vi "slow_control_2_12.vi"() -> ()   [LabVIEW 2018]
uses:
  4623b864-5764-45c6-9cb2-3e18237880ca.vi
  fa57f61f-0bb9-49ac-92eb-fcb40add4dbb.vi
  499f9cf5-7b15-41ea-951a-8da9be12721d.vi
  <vilib>/DAQmx/read.llb/DAQmx Read (Analog 1D DBL NChan 1Samp).vi
  ffb0d1b3-ef19-4e2e-b36e-7277177ef4b3.vi
  9a1acc8a-69db-4048-9e4c-bb07d66d2422.vi
  <vilib>/DAQmx/create/channels.llb/DAQmx Create Channel (AI-Voltage-Basic).vi
  <vilib>/DAQmx/create/channels.llb/DAQmx Create Channel (AI-Current-Basic).vi
  <vilib>/DAQmx/create/channels.llb/DAQmx Create Channel (AI-Temperature-RTD).vi
  <vilib>/DAQmx/miscellaneous.llb/DAQmx Fill In Error Info.vi
  <vilib>/Utility/file.llb/Read Delimited Spreadsheet (string).vi
  <instrlib>/Lake Shore 335/Lake Shore 335.lvlib
  <instrlib>/CAEN PSM/CAEN PSM.lvlib
  <resource>/objmgr/daqmx.rc
panel:
  out "Heater":dbl
  out "Coldhead":dbl
  out "Cycle number":i32
  out "Alarm state":bool
  out "Timestamp last \nmeasured (UPS)":timestamp
  out "Auto-clear":bool
  in  "Auto-clear data?":bool
  in  "Clear data":bool
  in  "Clear data every N cycles":dbl
  in  "N samples":i32=30
  out "Average Flow (SLPM)":dbl caption="Flow (SLPM)"
  out "CAEN Ch. Names":string[](array[string])
  in  "Cycles to execute":dbl=5.0 format="%#_13g"
  out "Detector Pressure":dbl
  in  "N samples":i32=20
  in  "Allows tabs on \nfront panel":T1(tab)
  in  "Specify up to six temperature sensors inside \nthe detector, separated with a comma.\nNumbers only, single commas!":string="10,11,12,13,14,15"
  out "Valid example:":string="11,12, 13, 15 ,14 "
  in  "Anode ch.":enum16{"1", "2", "3", "4"}(ring)=enum."3"
  in  "CAEN unit selector":enum16{"CAEN 1", "CAEN 2"}(ring)
  in  "Multipliers":dbl[](array[numeric])=[1.0, 1.0, 1.0, 1.0, 1.0, 1.0, 1.0, 1.0]
  in  "Offsets\nsubtracted":dbl[](array[numeric])=[0.0, 0.0, 0.0, 0.0, 0.0, 0.0, 0.0, 0.0]
  in  "Channel Names (9207, ai8:15)":string[](array[string])=["i0", "i1", "i2", "i3", "i4", "i5", "i6", "i7"] caption="\"Other\""
  in  "Flow meter input:":u16(ring)=3 items=["v0", "v1", "v2", "v3", "v4", "v5", "v6", "v7"]
  in  "Detector pressure input:":u16(ring) items=["v0", "v1", "v2", "v3", "v4", "v5", "v6", "v7"]
  in  "Channel Names (9207, ai0:7)":string[](array[string])=["v0", "v1", "v2", "v3", "v4", "v5", "v6", "v7"] caption="\"Other\""
  in  "Multipliers":dbl[](array[numeric])=[1.0, 1.0, 1.0, 1.0, 1.0, 1.0, 1.0, 1.0]
  in  "Offsets\nsubtracted":dbl[](array[numeric])=[0.0, 0.0, 0.0, 0.0, 0.0, 0.0, 0.0, 0.0]
  in  "Voltage channels":tag[](array[tag])=["9207/ai0", "9207/ai1", "9207/ai2", "9207/ai3", "9207/ai4", "9207/ai5", "9207/ai6", "9207/ai7"]
  in  "COM-port CAEN 1":refnum<visa-resource-name>
  in  "COM-port CAEN 2":refnum<visa-resource-name>
  in  "Run lakeshore?":bool
  in  "ID Query":bool
  in  "COM-port LakeShore":refnum<visa-resource-name>
  in  "PID settings":cluster{"P":dbl, "I":dbl, "D":dbl}={"P"=50.0, "I"=20.0, "D"=120.0}
  in  "Setpoint (°C)":dbl=-100.0 format="%.1f"
  in  "Heater range":u16(ring) items=["Off", "Low (On)", "Medium", "High"]
  in  "Current channels":tag[](array[tag])=["9207/ai8", "9207/ai9", "9207/ai10", "9207/ai11", "9207/ai12", "9207/ai13", "9207/ai14", "9207/ai15"]
  in  "Channel Names (CAEN)":string[](array[string])=["PMT 1", "PMT 2", "Anode", "Cathode", "Top gate", "Bottom gate", "Other 1", "Other 2"]
  in  "RTD Type":i32(ring)=10071 items=["Pt3750"=12481, "Pt3851"=10071, "Pt3911"=12482, "Pt3916"=10069, "Pt3920"=10053, "Pt3928"=12483, "Custom"=10137]
  in  "Module 1 channels (slot 1)":tag[](array[tag])=["cDAQ2Mod2/ai0", "cDAQ2Mod2/ai1", "cDAQ2Mod2/ai2", "cDAQ2Mod2/ai3", "cDAQ2Mod2/ai4", "cDAQ2Mod2/ai5", "cDAQ2Mod2/ai6", "cDAQ2Mod2/ai7"]
  in  "Current Excitation Source":i32(ring)=10200 items=["Internal"=10200, "External"=10167, "None"=10230]
  in  "Resistance Configuration":i32(ring)=3 items=["2-Wire"=2, "3-Wire"=3, "4-Wire"=4]
  in  "R (T = 0°C):":dbl=100.0
  in  "B":dbl
  in  "A":dbl
  in  "C":dbl
  in  "Module 2 channels (slot 2)":tag[](array[tag])=["cDAQ2Mod3/ai0", "cDAQ2Mod3/ai1", "cDAQ2Mod3/ai2", "cDAQ2Mod2/ai3", "cDAQ2Mod2/ai4", "cDAQ2Mod3/ai5", "cDAQ2Mod3/ai6", "cDAQ2Mod3/ai7"]
  in  "Shut off heater \nif Alarm is active":bool=TRUE
  in  "Re-save headers":bool
  in  "Resistance Configuration":i32(ring)=2 items=["2-Wire"=2, "3-Wire"=3, "4-Wire"=4]
  in  "Module 3 channels":tag[](array[tag])
  in  "RTD Type":i32(ring)=12481 items=["Pt3750"=12481, "Pt3851"=10071, "Pt3911"=12482, "Pt3916"=10069, "Pt3920"=10053, "Pt3928"=12483, "Custom"=10137]
  in  "R (T = 0°C)":dbl=100.0 format="%0.2f"
  out "PT1000 data":dbl[](array[numeric]) format="%0.2f"
  out "Det. T.":i32[](array[numeric])
  out "9207 (V; A) Converted":dbl[](array[numeric])
  out "9216 #1 (°C)":dbl[](array[numeric])
  out "9216 #2 (°C)":dbl[](array[numeric])
  out "Raw readouts (V, mA)":dbl[](array[numeric]) format="%0.2f"
  out "Det.P input #":i32
  out "Flow input #":i32
  out "PT100 data":dbl[](array[numeric]) format="%0.2f"
  in  "\"Sound\" alarm":bool
  in  "Sound alarm\nFrequency (Hz)":dbl=1680.0
  in  "Send status email now":bool
  out "Email error":i32
  out "source":string
  in  "Number of Bonus lines":i32=1
  out "Names (optional)":string[](array[string])
  in  "Send daily email?":bool=TRUE
  in  "Phone numbers":string[](array[string])
  out "Alarm (or test) message":string
  in  "Alarm\nMaster switch":bool
  in  "Repeat Alarm SMS\nevery N minutes":dbl=15.0
  in  "Test alarm":bool
  out "Warning":bool
  in  "UPS":bool
  in  "UPS Voltage \nLower Threshold":dbl=220.0
  out "String 6":string
  out "String 5":string
  out "String 4":string
  out "String 3":string
  out "String 2":string
  out "String":string
  out "NI mod 2&3 status":bool
  in  "NI mod 2&3":bool
  in  "NI mod 1":bool
  in  "CAEN 2":bool
  in  "CAEN 1":bool
  in  "LakeShore":bool
  out "Det. P. warning":bool
  out "Boolean 6":bool
  out "Boolean 5":bool
  out "Boolean 4":bool
  out "Boolean 3":bool
  out "Boolean 2":bool
  out "Boolean":bool
  in  "T 6":bool
  in  "T 5":bool
  in  "T 4":bool
  in  "T 3":bool
  in  "T 2":bool
  in  "T 1":bool
  in  "Detector Pressure":bool
  in  "Overpressure threshold":dbl
  in  "Underpressure threshold":dbl
  out "Comm. status":bool
  in  "High Temp threshold":dbl format="%#_13g"
  in  "Low Temp threshold":dbl format="%#_13g"
  out "LakeShore status":bool
  out "NI mod1 (P) status":bool
  out "CAEN 1 status":bool
  out "CAEN 2 status":bool
  out "Initialization status":bool
  out "Minimum input voltage measured":dbl
  out "Alarm active 2":bool
  out "SMS error":string
  out "Status email preview":string
  in  "Send status email at time:":string="14:00"
  in  "Email Addresses":string[](array[string])
  in  "return address":string="xamsups@gmail.com"
  in  "Ignore Initialization Errors":bool=TRUE caption="Ignore init. errors?"
  out "NI 9226":errorcluster
  in  "HV Channel status":string="Click the button to request the latest High Voltage channel status."
  out "CAEN 1":T2(array[cluster])
  out "CAEN 2":T2(array[cluster])
  in  "Query HV status":bool
  in  "\"code\"":string
  in  "String 7":string
  out "\"status\"":bool
  in  "\"source\"":string
  out "NI 9216 x2":errorcluster
  out "CAEN 1":errorcluster
  out "CAEN 2":errorcluster
  out "Lakeshore":errorcluster
  out "NI 9207":errorcluster
  out "9207 (ai 8:15, Amperes)":cluster{timestamp[], dbl[]}[](graph)
  in  "Temperature channel selector":u16(ring)=10 items=["10"=10, "11"=11, "12"=12, "13"=13, "14"=14, "15"=15, "Average"=666]
  out "Heater power (%)":cluster{timestamp[], dbl[]}[](graph)
  out "Flow (SLPM)":cluster{timestamp[], dbl[]}[](graph)
  out "9207 (ai 0:7, Volts)":cluster{timestamp[], dbl[]}[](graph)
  out "Phase Diagram":cluster{"X":dbl, "Y":dbl}[](graph)
  out "Temperature (ai 0:15, °C)":cluster{timestamp[], dbl[]}[](graph)
  in  "Pause?":bool
  out "Integrated Flow (SL)":dbl
  in  "Reset?":bool
  out "LakeShore readings":dbl[](array[numeric])
  out "Temp A":dbl
  out "Temp B":dbl
  in  "Temperature Channel Selector":u16(ring) items=["10"=10, "11"=11, "12"=12, "13"=13, "14"=14, "15"=15]
  out "Historical Large Phase Diagram":cluster{dbl[], dbl[]}[](graph)
  out "Large Phase Diagram":cluster{"X":dbl, "Y":dbl}[](graph)
  in  "Temperature Channel Selector":u16(ring)=666 items=["10"=10, "11"=11, "12"=12, "13"=13, "14"=14, "15"=15, "Average"=666]
  in  "Scale.Range:Minimum 8":dbl
  in  "Scale.Range:Maximum 8":dbl=4000.0
  in  "Scale.Range:Minimum 7":dbl
  in  "Scale.Range:Maximum 7":dbl=4000.0
  in  "Scale.Range:Minimum 6":dbl=-3000.0
  in  "Scale.Range:Maximum 6":dbl
  in  "Scale.Range:Minimum 5":dbl
  in  "Scale.Range:Maximum 5":dbl=3000.0
  in  "Scale.Range:Minimum 4":dbl=-5000.0
  in  "Scale.Range:Maximum 4":dbl
  in  "Scale.Range:Maximum 3":dbl=4000.0
  in  "Scale.Range:Minimum 3":dbl
  in  "Scale.Range:Maximum 2":dbl=1000.0
  in  "Scale.Range:Minimum 2":dbl
  out "CAEN 1.1":dbl(knob) scale=0.0..1000.0
  out "CAEN 1.1":string
  in  "Scale.Range:Maximum":dbl=1000.0
  in  "Scale.Range:Minimum":dbl
  out "CAEN 2.3 2":string
  out "CAEN 2.2 2":string
  out "Channel Names":string[](array[string])
  out "CAEN 2.3":dbl(knob) scale=0.0..4000.0
  out "CAEN 2.2":dbl(knob) scale=0.0..4000.0
  out "CAEN 2.1":string
  out "CAEN 2.0":string
  out "CAEN 1.3":string
  out "CAEN 1.2":string
  out "CAEN 1.0":string
  out "Channel Names":string[](array[string])
  in  "Set to zero":bool
  out "CAEN 2.1":dbl(knob)
  out "CAEN 2.0":dbl(knob) scale=0.0..3000.0
  in  "Apply Voltage":bool
  in  "VSet (V)":dbl[](array[numeric])
  in  "IMax (uA)":dbl[](array[numeric])
  in  "VMax (V)":dbl[](array[numeric])
  out "CAEN 1.3":dbl(knob)
  out "CAEN 1.2":dbl(knob) scale=0.0..4000.0
  out "CAEN 1.0":dbl(knob) scale=0.0..1000.0
  out "Vmon (V)":dbl[](array[numeric])
  out "IMon (uA)":dbl[](array[numeric])
  in  "Read CAEN units \nevery N cycles":i16=120
  in  "Reset anode\nperiodically?":bool
  in  "Kill every Y minutes":i32=10
  in  "Keep off for X seconds":i32=10
  out "?":bool
  out "Killed":bool
  out "Restarted":bool
  out "Anode timers":timestamp[](array[timestamp])
  out "Seconds until \nanode autokill":dbl format="%.2g"
  out "Seconds until \nanode reset":dbl format="%.2g"
  in  "Kill voltage":bool
  in  "stop":bool
  out "Voltages":dbl[](array[numeric])
  out "Started up?":bool
  out "TOBA appended":dbl[][](array[numeric])
  in  "Read T every N cycles":i32=2
  out "Time until next cycle":dbl format="%.3g"
  in  "Time per cycle (s)":i32=2 caption="Time Target (s)"
  # "<- Proof of concept for New/Old T + New P"
  # "Moving averages"
  # "NI 9216 Temperature settings"
  # "CAEN settings"
  # "NI 9207 Voltage settings"
  # "If RTD type is custom,\nspecify the Callendar-\nVan Dusen parameters"
  # "Anode connected to:"
  # "Channel:"
  # "NI 9207 Current settings"
  # "Lakeshore settings"
  # "NI 9226 Temperature settings"
  # "Gain (P) (XX.X)"
  # "Reset (I) (XX.X)"
  # "Rate (D) (X.X%)"
  # "Alarm indicators and arms"
  # "Detector Thresholds"
  # "Daily status email"
  # "SMS and sound alarm"
  # "Alarm conditions"
  # "Temperature channels:"
  # "Uninterruptable Power Supply"
  # "Device information"
  # "High Voltage channel status"
  # "How-to"
  # "Data"
  # "Scale:"
  # "to"
  # "to"
  # "Scale:"
  # "Time of last reset"
  # "Time of last reactivation"
  # "to"
  # "Scale:"
  # "to"
  # "Scale:"
  # "Settings"
  # "Scale:"
  # "to"
  # "Scale:"
  # "to"
  # "Scale:"
  # "to"
  # "to"
  # "Scale:"
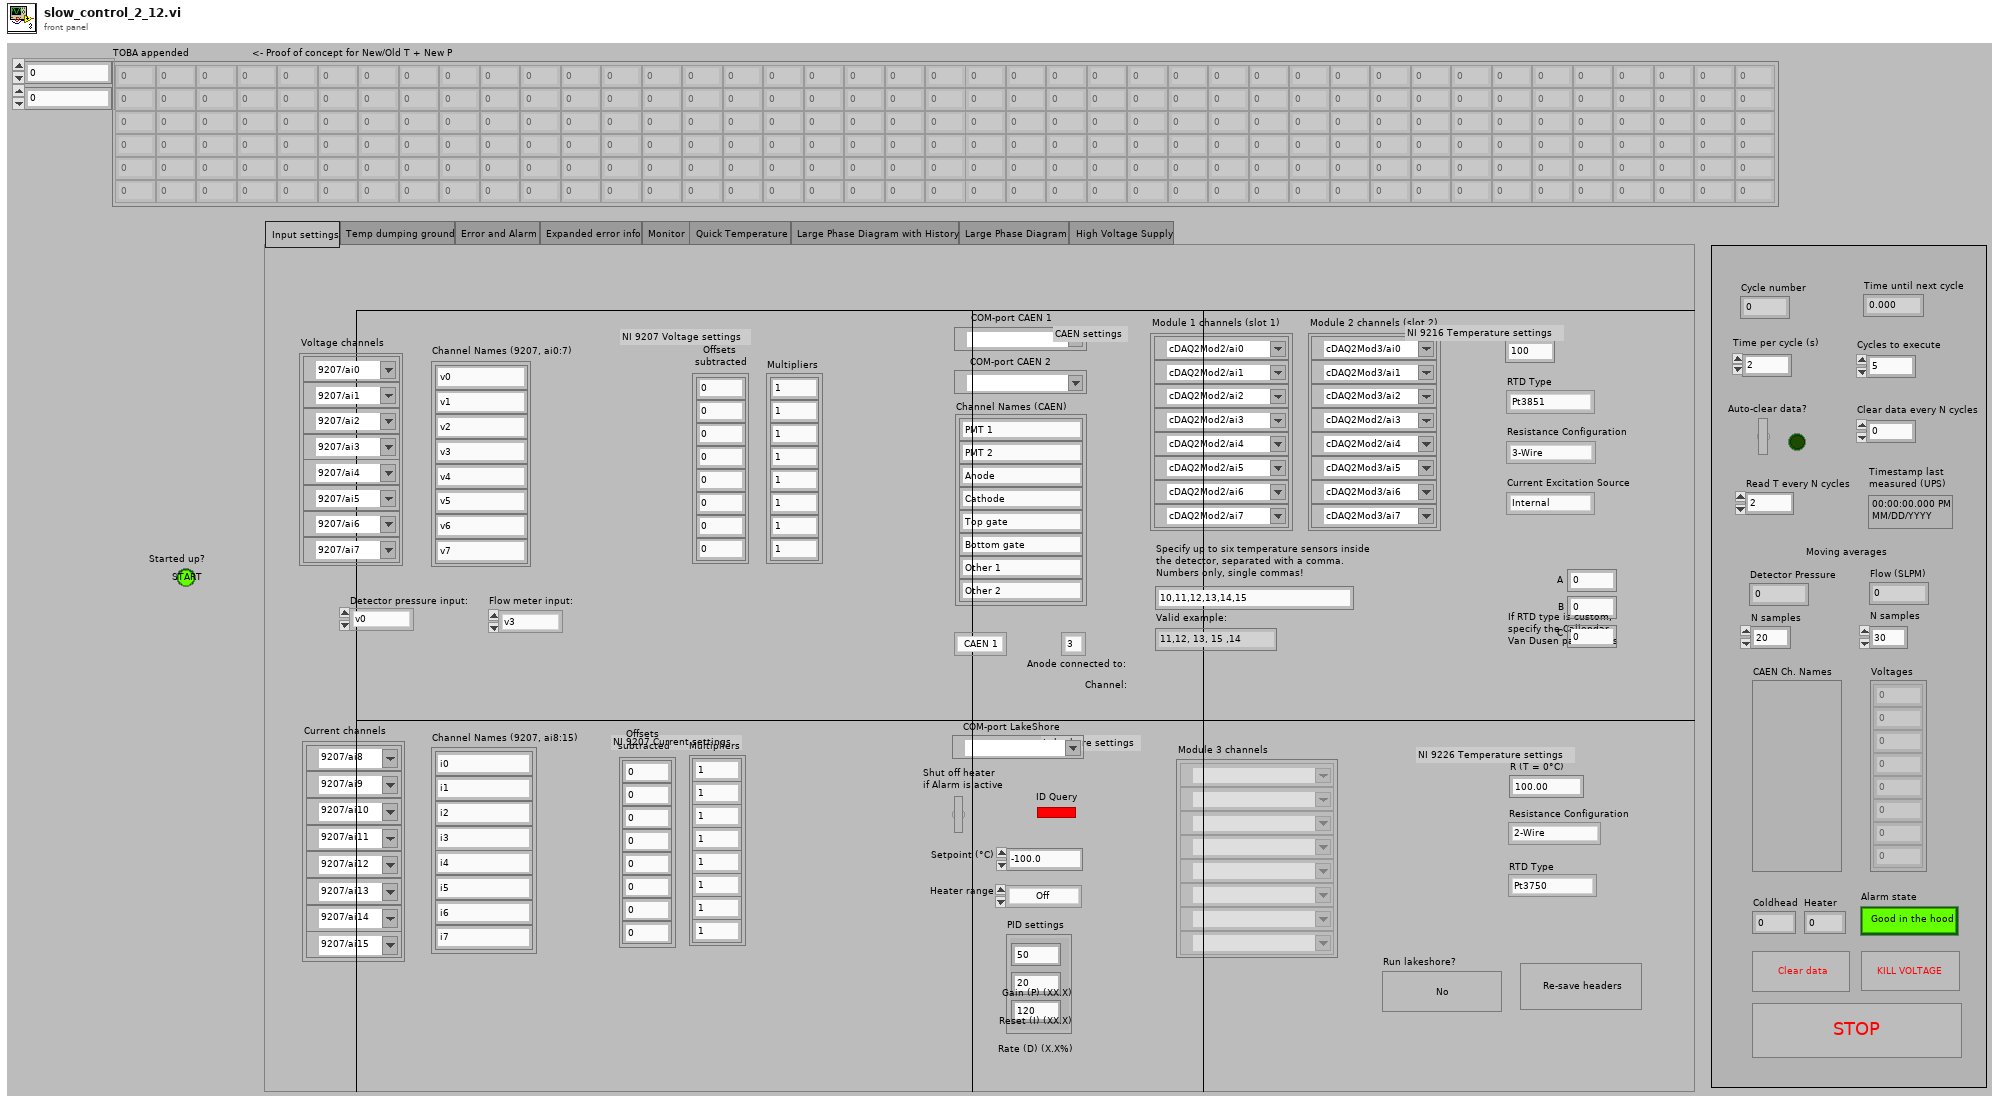
[diagram p1: front panel]
types:
  T1 = enum32{"Input settings", "Temp dumping ground", "Error and Alarm", "Expanded error info", "Monitor", "Quick Temperature", "Large Phase Diagram with History", "Large Phase Diagram", "High Voltage Supply"}
  T2 = cluster{"ON":bool, "RUP":bool, "RDW":bool, "OVC":bool, "OVV":bool, "UNV":bool, "MAXV":bool, "TRIP":bool, "OVP":bool, "OVT":bool, "DIS":bool, "KILL":bool, "ILK":bool, "NOCAL":bool}[]
  T3 = cluster{"Baud Rate":u32, "Parity":u16, "Data Bits":u16, "Stop Bits":u16, "Flow Control":u16}
  T4 = cluster{"task out":refnum<k21>, "error out":errorcluster}
  T5 = cluster{"VISA resource name out":refnum<visa-resource-name>, "error out":errorcluster}
  T6 = cluster{"VISA resource name out":refnum<visa-resource-name>, "Board address":u8, "NChannels":u8}
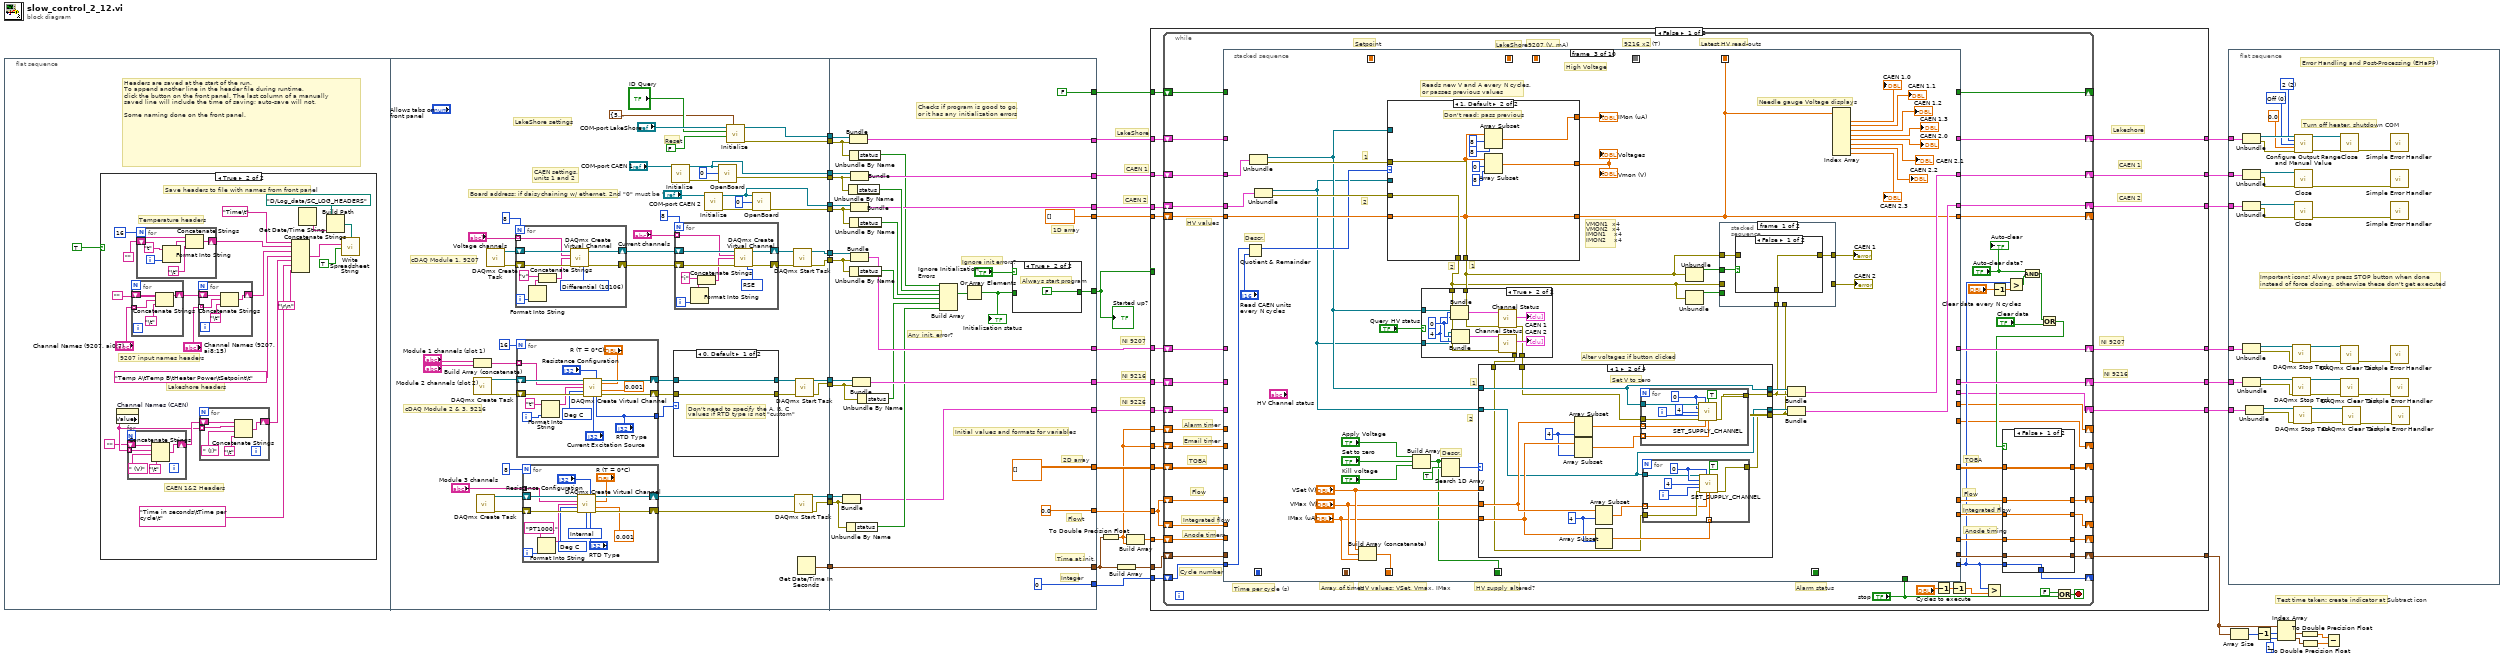
[diagram p0: block diagram]
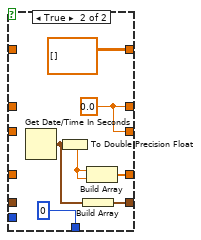
[diagram p2: hidden frame]
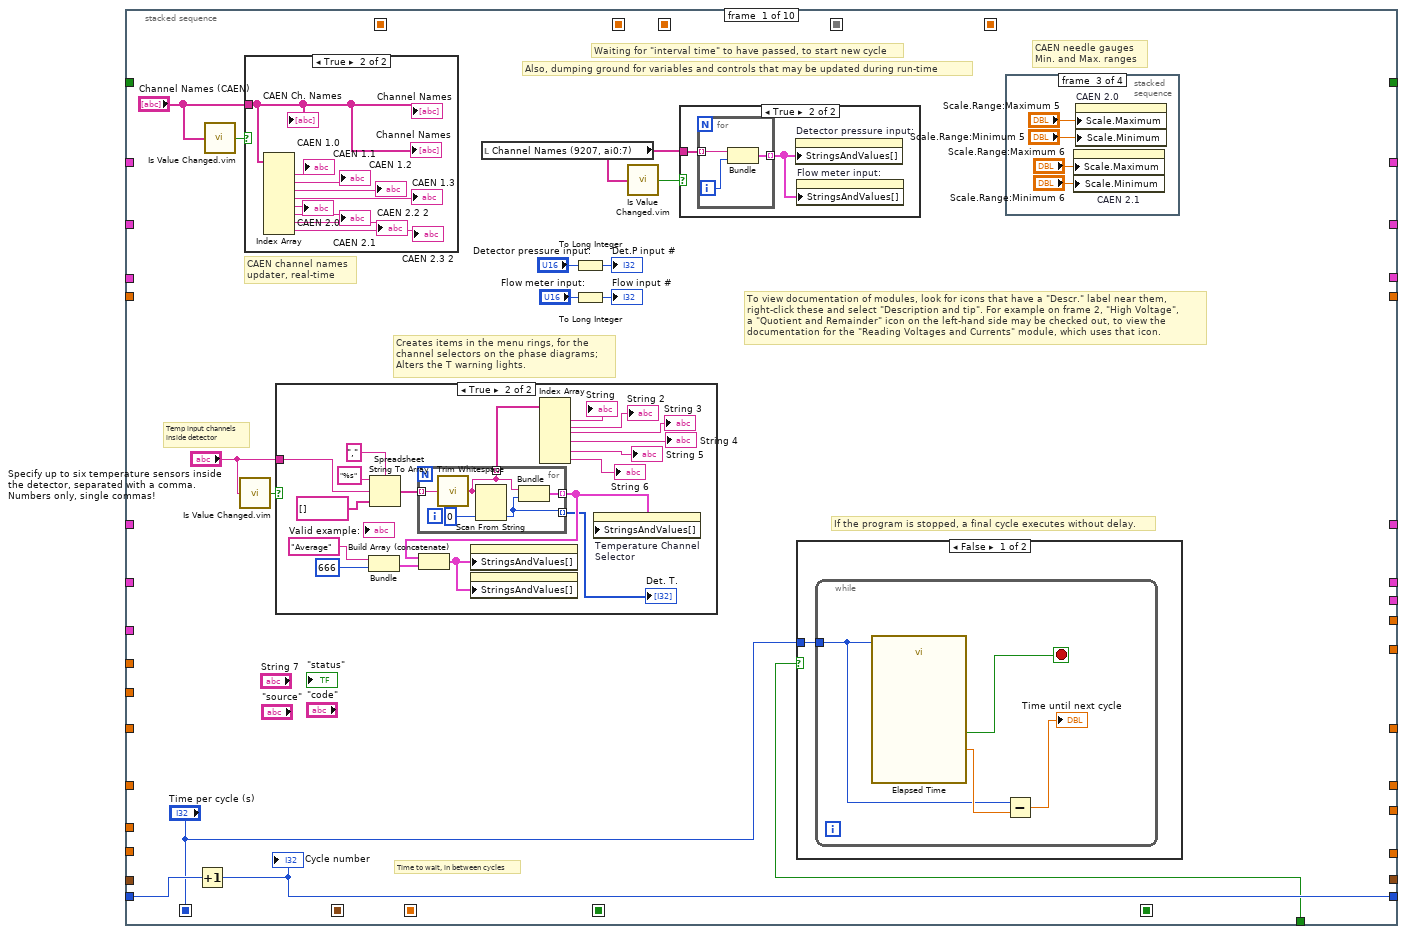
[diagram p3: hidden frame]
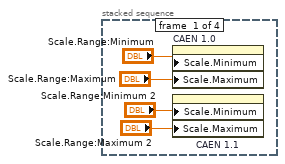
[diagram p7: hidden frame]
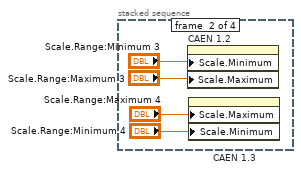
[diagram p8: hidden frame]
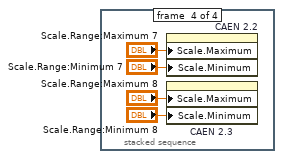
[diagram p9: hidden frame]
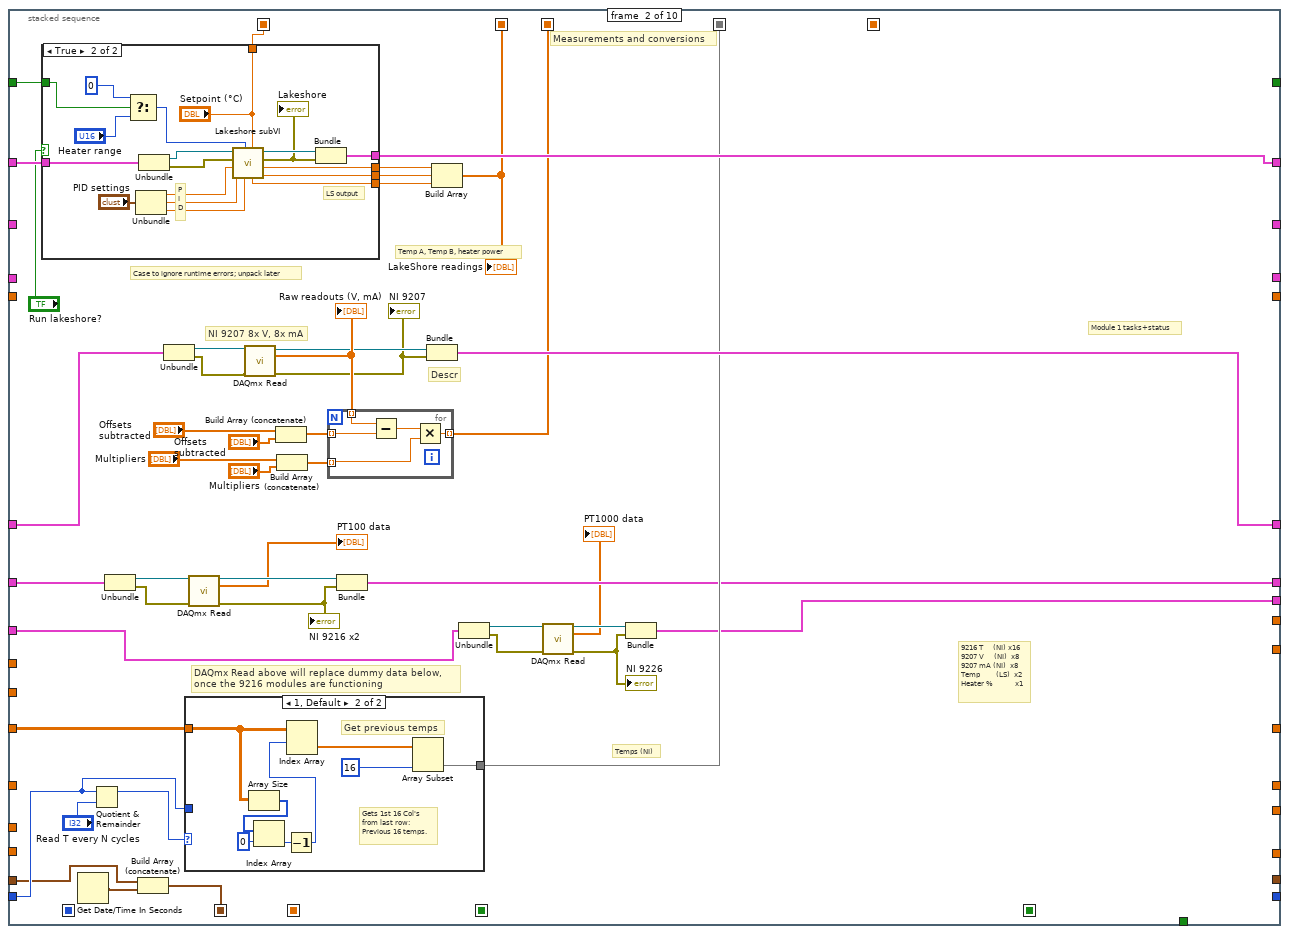
[diagram p11: hidden frame]
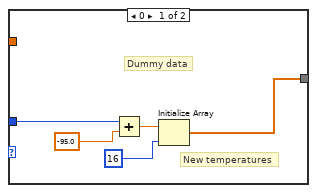
[diagram p12: hidden frame]
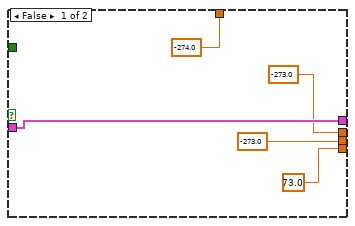
[diagram p13: hidden frame]
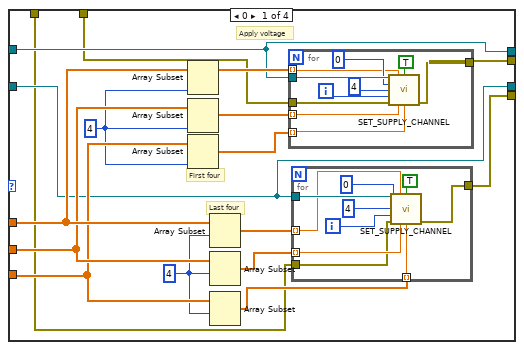
[diagram p18: hidden frame]
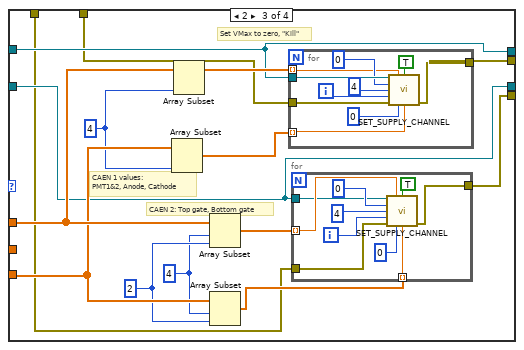
[diagram p19: hidden frame]
diagram:
  # "NI 9226"
  # "NI 9216"
  # "Test time taken: create indicator at Subtract icon"
  # "NI 9207"
  # "CAEN 2"
  # "CAEN 1"
  # "LakeShore"
  n1 = flat-sequence {
    tunnel: [w136] -> w43
    tunnel: [w135] -> w42
    tunnel: [w123] -> w41
    tunnel: [w132] -> w40
    tunnel: [w113] -> w39
    tunnel: [w131] -> w34
    tunnel: [w127] -> w26
    tunnel: [w126] -> w25
    tunnel: [w114] -> w17
    tunnel: [w108] -> w9
    tunnel: [w107] -> w8
    tunnel: [w91] -> w4
    tunnel: [w90] -> w3
    tunnel: w43 -> [w227]
    tunnel: w42 -> [w226]
    tunnel: w41 -> [w224]
    tunnel: w40 -> [w223]
    tunnel: w39 -> [w213]
    tunnel: [w228] -> w23
    tunnel: [0.0] -> w22
    tunnel: [dbl[] []] -> w38
    tunnel: [dbl[][] []] -> w10
    tunnel: [0] -> w37
    tunnel: [w225] -> w36
    tunnel: [w222] -> w35
    tunnel: [w221] -> w21
    tunnel: w34 -> [w221]
    tunnel: w26 -> [w219]
    tunnel: w25 -> [w218]
    tunnel: [w217] -> w24
    tunnel: [FALSE] -> w18
    tunnel: w17 -> [w214]
    tunnel: [w212] -> w16
    tunnel: w9 -> [w205]
    tunnel: w8 -> [w204]
    tunnel: [w203] -> w7
    tunnel: w4 -> [w200]
    tunnel: w3 -> [w199]
    tunnel: [w197] -> w2
    frame #0 {
      # "Headers are saved at the start of the run.\nTo append another line in the header file during runtime,\nclick the button on the front panel. The last column of a manually\nsaved line will include the time of saving; auto-save will not.\n\nSome naming done on the front panel."
      n2 = case shown="True" TRUE {
        frame False {
        }
        frame True {
          # "CAEN 1&2 Headers"
          # "Lakeshore headers"
          # "9207 input names headers"
          # "Temperature headers"
          # "Save headers to file with names from front panel"
          n3 = property on="Channel Names (CAEN)" class="Arr (strict)"() -> ("Value"=w50:string[])  [unwired: 2 in, 2 out]
          n4 = for {
            tunnel: w50 -> [w74] mode=indexing
            shift-right: [w72] -> w51
            shift-left: "" -> [w71]
            n5 = Concatenate Strings(w71, w74, " (V)", "\t") -> (w72:string)
          }
          n6 = for {
            shift-right: [w82] -> w54
            shift-left: "" -> [w83]
            tunnel: "Channel Names (9207, ai0:7)" -> [w80] mode=indexing
            n7 = Concatenate Strings(w83, w80, "\t") -> (w82:string)
          }
          n8 = for {
            N: 16 -> [_]
            shift-right: [w84] -> w57
            shift-left: "" -> [w85]
            i -> [w89]
            n9 = Format Into String(initial string="t", w89) -> (resulting string=w87:string)  [unwired: 2 in, 1 out]
            n10 = Concatenate Strings(w85, w87, "\t") -> (w84:string)
          }
          n11 = for {
            shift-right: [w77] -> w53
            shift-left: w54 -> [w79]
            tunnel: "Channel Names (9207, ai8:15)" -> [w76] mode=indexing
            n12 = Concatenate Strings(w79, w76, "\t") -> (w77:string)
          }
          n13 = for {
            shift-right: [w67] -> w49
            shift-left: w51 -> [w68]
            tunnel: w50 -> [w66] mode=indexing
            n14 = Concatenate Strings(w68, w66, " (I)", "\t") -> (w67:string)
          }
          n15 = Concatenate Strings("Time\t", w57, w53, "Temp A\tTemp B\tHeater Power\tSetpoint\t", w49, "Time in seconds\tTime per cycle\t", "\r\n") -> (w56:string)
          n16 = Get Date/Time String() -> (date string=w60:string)  [unwired: 3 in, 1 out]
          n17 = Build Path(base path=path "D:/Log_data/SC_LOG_HEADERS" ("file path (dialog if empty)"), name or relative path=w60) -> (appended path=w61:path)
          n18 = call <vilib>:"Write Spreadsheet String.vi"("append to file? (new file:F)"=TRUE, "spreadsheet string"=w56, "file path (dialog if empty)"=w61) -> ()  [unwired: 7 in, 2 out]
        }
      }
    }
    frame #1 {
      # "cDAQ Module 2 & 3, 9216"
      # "cDAQ Module 1, 9207"
      # "Board address: if daisychaining w/ ethernet, 2nd \"0\" must be \"1\""
      # "CAEN settings,\nunits 1 and 2"
      # "Reset"
      # "LakeShore settings"
      n19 = call <vilib>:"DAQmx Create Task.vi"() -> ("task out"=w106:refnum<k21>, "error out"=w109:errorcluster)  [unwired: 14 in]
      n20 = Build Array (concatenate)("Module 1 channels (slot 1)", "Module 2 channels (slot 2)") -> (w103:tag[])
      n21 = call <vilib>:"DAQmx Create Task.vi"() -> ("task out"=w96:refnum<k21>, "error out"=w95:errorcluster)  [unwired: 14 in]
      n22 = call <vilib>:"DAQmx Create Task.vi"() -> ("task out"=w122:refnum<k21>, "error out"=w121:errorcluster)  [unwired: 14 in]
      n23 = for {
        N: 8 -> [_]
        shift-right: [w192] -> w118
        shift-left: w122 -> [w191]
        shift-right: [w193] -> w117
        shift-left: w121 -> [w189]
        tunnel: "Voltage channels" -> [w190] mode=indexing
        i -> [w195]
        w187 = 10106 items=["Default"=-1, "RSE"=10083, "NRSE"=10078, "Differential"=10106, "Pseudodifferential"=12529] ("input terminal configuration")
        n24 = Format Into String(w195) -> (resulting string=w194:string)  [unwired: 3 in, 1 out]
        n25 = Concatenate Strings("v" ("string"), w194) -> (w188:string)
        n26 = call-poly <vilib>:"DAQmx Create Virtual Channel.vi"("task in"=w191, "input terminal configuration"=w187, "physical channels"=w190, "name to assign"=w188, "error in"=w189) -> ("task out"=w192:refnum<k21>, "error out"=w193:errorcluster)  [unwired: 9 in]
      }
      n27 = for {
        N: 16 -> [_]
        shift-right: [w173] -> w102
        shift-left: w106 -> [w176]
        shift-right: [w174] -> w101
        shift-left: w109 -> [w175]
        tunnel: w103 -> [w172] mode=indexing
        tunnel: ["RTD Type"] -> w98
        i -> [w170]
        w167 = 10143 items=["Deg C"=10143, "Deg F"=10144, "Kelvins"=10325, "Deg R"=10145, "From Custom Scale"=10065] ("units")
        n28 = Format Into String(initial string="t", w170) -> (resulting string=w169:string)  [unwired: 2 in, 1 out]
        n29 = call-poly <vilib>:"DAQmx Create Virtual Channel.vi"("task in"=w176, "resistance configuration"="Resistance Configuration", "physical channels"=w172, "r0"="R (T = 0°C):", "name to assign"=w169, "units"=w167, "current excitation value"=0.001, "error in"=w175, "current excitation source"="Current Excitation Source", "rtd type"="RTD Type") -> ("task out"=w173:refnum<k21>, "error out"=w174:errorcluster)  [unwired: 4 in]
      }
      n30 = for {
        N: 8 -> [_]
        shift-right: [w151] -> w93
        shift-left: w96 -> [w150]
        shift-right: [w152] -> w92
        shift-left: w95 -> [w153]
        tunnel: "Module 3 channels" -> [w148] mode=indexing
        i -> [w146]
        w142 = 10200 items=["Internal"=10200, "External"=10167, "None"=10230] ("current excitation source")
        w144 = 10143 items=["Deg C"=10143, "Deg F"=10144, "Kelvins"=10325, "Deg R"=10145, "From Custom Scale"=10065] ("units")
        n31 = Format Into String(initial string="PT1000.", w146) -> (resulting string=w145:string)  [unwired: 2 in, 1 out]
        n32 = call-poly <vilib>:"DAQmx Create Virtual Channel.vi"("task in"=w150, "resistance configuration"="Resistance Configuration", "physical channels"=w148, "r0"="R (T = 0°C)", "name to assign"=w145, "units"=w144, "current excitation value"=0.001, "error in"=w153, "current excitation source"=w142, "rtd type"="RTD Type") -> ("task out"=w151:refnum<k21>, "error out"=w152:errorcluster)  [unwired: 4 in]
      }
      n33 = call <instrlib>:"Initialize.vi"("VISA resource name"="COM-port CAEN 1") -> ("error out"=w133:errorcluster, "VISA resource name out"=w123:refnum<visa-resource-name>)  [unwired: 9 in]
      n34 = case shown="0, Default" w98 {
        tunnel: w102 -> [w155 w159]
        tunnel: w101 -> [w154 w158]
        tunnel: [w155 w157] -> w100
        tunnel: [w154 w156] -> w99
        frame 0, Default {
          # "Don't need to specify the A, B, C\nvalues if RTD type is not \"custom\""
        }
        frame 10137 {
          # "RTD type =  \"custom\""
          n35 = property class="DAQmx Channel"(reference=w159, error in=w158, "AI.RTD.A"="A", "AI.RTD.B"="B", "AI.RTD.C"="C") -> (reference out=w157:refnum<k21>, error out=w156:errorcluster)
        }
      }
      n36 = for {
        N: 8 -> [_]
        shift-right: [w178] -> w115
        shift-left: w118 -> [w185]
        shift-right: [w177] -> w116
        shift-left: w117 -> [w184]
        tunnel: "Current channels" -> [w183] mode=indexing
        i -> [w182]
        w186 = 10083 items=["default"=-1, "RSE"=10083, "NRSE"=10078, "Differential"=10106, "Pseudodifferential"=12529] ("input terminal configuration")
        n37 = Format Into String(w182) -> (resulting string=w180:string)  [unwired: 3 in, 1 out]
        n38 = Concatenate Strings("i", w180) -> (w179:string)
        n39 = call-poly <vilib>:"DAQmx Create Virtual Channel.vi"("task in"=w185, "input terminal configuration"=w186, "physical channels"=w183, "name to assign"=w179, "error in"=w184) -> ("task out"=w178:refnum<k21>, "error out"=w177:errorcluster)  [unwired: 9 in]
      }
      n40 = call <instrlib>:"Initialize.vi"("VISA resource name"="COM-port CAEN 2") -> ("error out"=w128:errorcluster, "VISA resource name out"=w127:refnum<visa-resource-name>)  [unwired: 9 in]
      n41 = call <instrlib>:"OpenBoard.vi"("error in (no error)"=w133, "Board Address"=0, "VISA resource name"=w123) -> ("error out"=w132:errorcluster)  [unwired: 7 in, 1 out]
      n42 = call <instrlib>:"Initialize.vi"("Serial Configuration"=T3 {"Baud Rate"=57600, "Parity"=1, "Data Bits"=7, "Stop Bits"=10, "Flow Control"=0}, "Reset (True)"=FALSE ("Reset (LakeShore)"), "ID Query (True)"="ID Query", "VISA resource name"="COM-port LakeShore") -> ("error out"=w135:errorcluster, "VISA resource name out"=w136:refnum<visa-resource-name>)  [unwired: 6 in]
      n43 = call <instrlib>:"OpenBoard.vi"("error in (no error)"=w128, "Board Address"=u8 0, "VISA resource name"=w127) -> ("error out"=w126:errorcluster)  [unwired: 7 in, 1 out]
      n44 = call <vilib>:"DAQmx Start Task.vi"("task/channels in"=w115, "error in"=w116) -> ("task out"=w114:refnum<k21>, "error out"=w113:errorcluster)  [unwired: 12 in]
      n45 = call <vilib>:"DAQmx Start Task.vi"("task/channels in"=w93, "error in"=w92) -> ("task out"=w91:refnum<k21>, "error out"=w90:errorcluster)  [unwired: 12 in]
      n46 = call <vilib>:"DAQmx Start Task.vi"("task/channels in"=w100, "error in"=w99) -> ("task out"=w108:refnum<k21>, "error out"=w107:errorcluster)  [unwired: 12 in]
      n47 = Get Date/Time In Seconds() -> (seconds since 1Jan1904=w131:timestamp)
    }
    frame #2 {
      # "1D array"
      # "Initial values and formats for variables"
      # "Time at init."
      # "Integer"
      # "2D array"
      # "Flowt"
      # "Checks if program is good to go,\nor it has any initialization errors"
      # "Ignore init errors?"
      # "Any init. error?"
      n48 = Bundle("task out"=w200, "error out"=w199) -> (w197:T4)  [unwired: 1 in]
      n49 = Unbundle By Name(w199) -> ("status"=w198:bool)
      n50 = Unbundle By Name(w223) -> ("status"=w229:bool)
      n51 = Unbundle By Name(w226) -> ("status"=w206:bool)
      n52 = Bundle("VISA resource name out"=w227, "error out"=w226) -> (w225:T5)  [unwired: 1 in]
      n53 = Unbundle By Name(w218) -> ("status"=w220:bool)
      n54 = Unbundle By Name(w213) -> ("status"=w207:bool)
      n55 = Bundle("VISA resource name out"=w219, "error out"=w218) -> (w217:T5)  [unwired: 1 in]
      n56 = Bundle("task out"=w214, "error out"=w213) -> (w212:T4)  [unwired: 1 in]
      n57 = Bundle("VISA resource name out"=w224, "error out"=w223) -> (w222:T5)  [unwired: 1 in]
      n58 = Bundle("task out"=w205, "error out"=w204) -> (w203:T4)  [unwired: 1 in]
      n59 = Unbundle By Name(w204) -> ("status"=w202:bool)
      n60 = Build Array(w206, w229, w207, w220, w202, w198) -> (w230:bool[])
      n61 = Or Array Elements(Boolean array=w230) -> (logical OR=w201:bool)
      "Initialization status" <- w201
      n62 = case shown="True" "Ignore Initialization Errors" {
        tunnel: [w231 FALSE] -> w228
        tunnel: w201 -> [w231 _]
        frame False {
          # "Only start if no errors"
        }
        frame True {
          # "Always start program"
        }
      }
    }
  }
  n63 = To Double Precision Float(number=w21) -> (double precision float=w5:dbl)
  n64 = Build Array(w21) -> (w33:timestamp[])
  n65 = Build Array(w5, w5) -> (w20:dbl[])
  n66 = case shown="False" w23 {
    selector: w23 -> [_ w1191]
    tunnel: [_ w1191] -> _
    tunnel: w38 -> [w247 _]
    tunnel: w37 -> [w254 _]
    tunnel: w10 -> [w253 _]
    tunnel: w36 -> [w248 w1189]
    tunnel: w35 -> [w250 w1188]
    tunnel: w33 -> [w252 _]
    tunnel: [w251 timestamp[] []] -> w29
    tunnel: w24 -> [w249 w1187]
    tunnel: w22 -> [w243 _]
    tunnel: w20 -> [w246 _]
    tunnel: [w245 w1189] -> w19
    tunnel: w18 -> [w244 _]
    tunnel: w16 -> [w242 w1186]
    tunnel: [w241 w1188] -> w15
    tunnel: [w240 w1187] -> w14
    tunnel: [w239 w1186] -> w13
    tunnel: w7 -> [w238 w1185]
    tunnel: [w237 w1185] -> w6
    tunnel: w5 -> [w236 _]
    tunnel: w5 -> [w235 _]
    tunnel: w2 -> [w234 w1184]
    tunnel: [w233 w1184] -> w1
    frame False {
      # "NI 9216"
      # "NI 9207"
      # "CAEN 2"
      # "CAEN 1"
      # "Lakeshore"
      n67 = while {
        shift-right: [w267] -> _
        shift-left: w254 -> [w305]
        shift-right: [w280] -> _
        shift-left: w253 -> [w294]
        shift-right: [w272] -> w251
        shift-left: w252 -> [w302]
        shift-right: [w296] -> w241
        shift-left: w250 -> [w289]
        shift-right: [w298] -> _
        shift-left: w247 -> [w301]
        shift-right: [w295] -> w240
        shift-left: w249 -> [w300]
        shift-right: [w297] -> w245
        shift-left: w248 -> [w299]
        shift-right: [w276] -> _
        shift-left: w243 -> [w291]
        shift-right: [w278] -> _
        shift-left: w243 -> [w292]
        shift-right: [w274] -> _
        shift-left: w246 -> [w290]
        shift-right: [w262] -> _
        shift-left: w244 -> [w288]
        shift-right: [w286] -> w239
        shift-left: w242 -> [w287]
        shift-right: [w284] -> w237
        shift-left: w238 -> [w285]
        shift-right: [w260] -> _
        shift-left: w236 -> [w261]
        shift-right: [w257] -> _
        shift-left: w235 -> [w258]
        shift-right: [w255] -> w233
        shift-left: w234 -> [w256]
        stop <- w303 stop-if-true
        # "Email timer"
        # "Alarm timer"
        # "Alarm status"
        # "LakeShore"
        # "9216 x2 (T)"
        # "9207 (V, mA)"
        # "HV supply altered?"
        # "Setpoint"
        # "Anode timing"
        # "Anode timers"
        # "Integrated flow"
        # "Flow"
        # "Flow"
        # "Integrated Flow"
        # "TOBA"
        # "Array of times"
        # "Latest HV read-outs"
        # "Time per cycle (s)"
        # "Cycle number"
        # "HV values: VSet, Vmax, IMax"
        # "HV values"
        # "TOBA"
        n68 = stacked-sequence {
          seq-local: [_ _ w499 _ _ _ _ _ _ _] -> [_ _ _ w689 _ _ _ _ _ _]
          seq-local: ["Time per cycle (s)" _ _ _ _ _ _ _ _ _] -> [_ _ _ _ _ _ w882 _ _ _]
          seq-local: [_ _ w490 _ _ _ _ _ _ _] -> [_ _ _ _ _ _ w884 _ _ _]
          seq-local: [_ w431 _ _ _ _ _ _ _ _] -> [_ _ _ _ w761 w870 _ _ _ _]
          seq-local: [_ _ w493 _ _ _ _ _ _ _] -> [_ _ _ w684 _ _ _ _ _ _]
          seq-local: [_ w424 _ _ _ _ _ _ _ _] -> [_ _ _ _ _ _ w899 _ _ _]
          seq-local: [_ w419 _ _ _ _ _ _ _ _] -> [_ _ _ _ w799 w862 w886 w987 w1022 w1109]
          seq-local: [_ w418 _ _ _ _ _ _ _ _] -> [_ _ _ _ w790 w865 w887 w988 w1021 w1111]
          seq-local: [_ w406 _ _ _ _ _ _ _ _] -> [_ _ _ _ w797 w864 w885 _ _ _]
          seq-local: [_ _ _ _ _ _ _ w947 _ _] -> [_ _ _ _ _ _ _ _ w1024 w1110]
          tunnel: [w331 _ _ _ _ _ _ _ _ _] -> w266
          tunnel: "stop" -> [w330 _ _ _ _ _ _ _ _ _]
          tunnel: w305 -> [w332 w420 w515 _ _ _ _ _ _ _]
          tunnel: w294 -> [_ w421 _ _ w800 _ _ _ _ _]
          tunnel: [_ _ _ _ w777 _ _ _ _ _] -> w281
          tunnel: w302 -> [_ w398 _ _ _ _ _ _ _ _]
          tunnel: w289 -> [_ _ w522 w690 _ _ _ w1004 _ _]
          tunnel: w301 -> [_ _ w520 _ _ _ _ _ _ _]
          tunnel: w300 -> [_ _ w519 w685 _ _ _ w1003 _ _]
          tunnel: w299 -> [_ w433 _ _ _ _ _ w1002 _ _]
          tunnel: [_ w434 _ _ _ _ _ _ _ _] -> w297
          tunnel: [_ _ w490 _ _ _ _ _ _ _] -> w298
          tunnel: [_ _ w505 _ _ _ _ _ _ _] -> w296
          tunnel: [_ _ w503 _ _ _ _ _ _ _] -> w295
          tunnel: [_ _ _ _ w761 _ _ _ _ _] -> w273
          tunnel: w291 -> [_ _ _ _ _ w868 _ _ _ _]
          tunnel: w292 -> [_ _ _ _ _ w869 _ _ _ _]
          tunnel: w290 -> [_ _ _ w691 _ _ _ _ _ _]
          tunnel: [_ _ _ w686 _ _ _ _ _ _] -> w275
          tunnel: w288 -> [_ w427 _ _ _ _ _ _ _ _]
          tunnel: w287 -> [_ w426 _ _ _ _ _ w1001 _ _]
          tunnel: [_ w422 _ _ _ _ _ _ _ _] -> w286
          tunnel: [_ _ _ _ _ w867 _ _ _ _] -> w277
          tunnel: [_ _ _ _ _ w866 _ _ _ _] -> w279
          tunnel: w285 -> [_ w405 _ _ _ _ _ w989 _ _]
          tunnel: [_ w400 _ _ _ _ _ _ _ _] -> w284
          tunnel: [_ _ _ _ _ _ _ _ w1026 _] -> w262
          tunnel: w261 -> [_ _ _ _ _ _ _ _ w1020 _]
          tunnel: [_ _ _ _ _ _ _ _ w1018 _] -> w260
          tunnel: w258 -> [_ _ _ _ _ _ _ _ _ w1097]
          tunnel: [_ _ _ _ _ _ _ _ _ w1096] -> w257
          tunnel: w256 -> [_ w397 _ _ _ _ _ _ _ _]
          tunnel: [_ w392 _ _ _ _ _ _ _ _] -> w255
          frame #0 {
            # "Temp input channels\ninside detector"
            # "CAEN channel names\nupdater, real-time"
            # "Creates items in the menu rings, for the channel selectors on the phase diagrams;\nAlters the T warning lights."
            # "Also, dumping ground for variables and controls that may be updated during run-time"
            # "CAEN needle gauges\nMin. and Max. ranges"
            # "To view documentation of modules, look for icons that have a \"Descr.\" label near them,\nright-click these and select \"Description and tip\". For example on frame 2, \"High Voltage\",\na \"Quotient and Remainder\" icon on the left-hand side may be checked out, to view the\ndocumentation for the \"Reading Voltages and Currents\" module, which uses that icon."
            # "Time to wait, in between cycles"
            # "If the program is stopped, a final cycle executes without delay."
            # "Waiting for \"interval time\" to have passed, to start new cycle"
            n69 = Increment(x=w332) -> (x+1=w331:i32)
            "Cycle number" <- w331
            n70 = call "Is Value Changed.vim"("value"="Channel Names (CAEN)") -> ("changed or first call?"=w321:bool)
            n71 = call "Is Value Changed.vim"("value"="Specify up to six temperature sensors inside \nthe detector, separated with a comma.\nNumbers only, single commas!") -> ("changed or first call?"=w323:bool)
            n72 = case shown="True" w321 {
              tunnel: "Channel Names (CAEN)" -> [_ w338]
              frame False {
              }
              frame True {
                n73 = Index Array(array=w338) -> (element #1=→"CAEN 1.0":string, element #2=→"CAEN 1.1":string, element #3=→"CAEN 1.2":string, element #4=→"CAEN 1.3":string, element #5=→"CAEN 2.0":string, element #6=→"CAEN 2.1":string, element #7=→"CAEN 2.2 2":string, element #8=→"CAEN 2.3 2":string)  [unwired: 8 in]
                "CAEN Ch. Names" <- w338
                "Channel Names" <- w338
                "Channel Names" <- w338
              }
            }
            n74 = case shown="True" w323 {
              tunnel: "Specify up to six temperature sensors inside \nthe detector, separated with a comma.\nNumbers only, single commas!" -> [_ w348]
              frame False {
              }
              frame True {
                n75 = Bundle("Average", 666) -> (w354:cluster{string, i32})  [unwired: 1 in]
                n76 = Spreadsheet String To Array(delimiter (Tab)=",", format string="%s", spreadsheet string=w348, array type (2D Dbl)=string[] []) -> (array=w357:string[])
                n77 = for {
                  tunnel: w357 -> [w369] mode=indexing
                  tunnel: [w367] -> w356 mode=indexing
                  tunnel: [w366] -> w347 mode=indexing
                  tunnel: [w365] -> w358 mode=indexing
                  n78 = call <vilib>:"Trim Whitespace.vi"("string"=w369) -> ("trimmed string"=w365:string)  [unwired: 1 in]
                  n79 = Scan From String(input string=w365, default 1=0) -> (output 1=w366:i32)  [unwired: 3 in, 3 out]
                  n80 = Bundle("trimmed string"=w365, w366) -> (w367:cluster{"trimmed string":string, i32})  [unwired: 1 in]
                }
                "Det. T." <- w347
                n81 = Build Array (concatenate)(w356, w354) -> (w355:cluster{"trimmed string":string, i32}[])
                n82 = property on="Temperature channel selector" class="Ring (strict)"("StringsAndValues[]"=w355) -> ()  [unwired: 2 in, 2 out]
                n83 = property on="Temperature Channel Selector" class="Ring (strict)"("StringsAndValues[]"=w355) -> ()  [unwired: 2 in, 2 out]
                n84 = Index Array(array=w358) -> (element #1=→"String":string, element #2=→"String 2":string, element #3=→"String 3":string, element #4=→"String 4":string, element #5=→"String 5":string, element #6=→"String 6":string)  [unwired: 6 in]
                n85 = property on="Temperature Channel Selector" class="Ring (strict)"("StringsAndValues[]"=w356) -> ()  [unwired: 2 in, 2 out]
              }
            }
            n86 = local read "Channel Names (9207, ai0:7)"() -> (w319:string[])
            n87 = To Long Integer(number="Detector pressure input:") -> (32bit integer=→"Det.P input #":i32)
            n88 = To Long Integer(number="Flow meter input:") -> (32bit integer=→"Flow input #":i32)
            n89 = call "Is Value Changed.vim"("value"=w319) -> ("changed or first call?"=w320:bool)
            n90 = case shown="True" w320 {
              tunnel: w319 -> [_ w334]
              frame False {
                # ":D"
              }
              frame True {
                n91 = for {
                  tunnel: w334 -> [w337] mode=indexing
                  tunnel: [w335] -> w333 mode=indexing
                  i -> [w336]
                  n92 = Bundle("Or give name if \"Other\""=w337, w336) -> (w335:cluster{"Or give name if \"Other\"":string, i32})  [unwired: 1 in]
                }
                n93 = property on="Detector pressure input:" class="Ring (strict)"("StringsAndValues[]"=w333) -> ()  [unwired: 2 in, 2 out]
                n94 = property on="Flow meter input:" class="Ring (strict)"("StringsAndValues[]"=w333) -> ()  [unwired: 2 in, 2 out]
              }
            }
            n95 = case shown="False" w330 {
              tunnel: "Time per cycle (s)" -> [w386 _]
              frame False {
                n96 = while {
                  tunnel: w386 -> [w388]
                  stop <- w390 stop-if-true
                  n97 = call "Elapsed Time"("Time Target (s)"=w388) -> ("Elapsed Time (s)"=w389:dbl, "Time has Elapsed"=w390:bool)  [unwired: 11 in, 6 out]
                  n98 = Subtract(x=w388, y=w389) -> (x-y=→"Time until next cycle":dbl)
                }
              }
              frame True {
              }
            }
            n99 = stacked-sequence {
              frame #0 {
                n100 = property on="CAEN 1.0" class="Knob (strict)"("Scale.Minimum"="Scale.Range:Minimum", "Scale.Maximum"="Scale.Range:Maximum") -> ()  [unwired: 2 in, 2 out]
                n101 = property on="CAEN 1.1" class="Knob (strict)"("Scale.Minimum"="Scale.Range:Minimum 2", "Scale.Maximum"="Scale.Range:Maximum 2") -> ()  [unwired: 2 in, 2 out]
              }
              frame #1 {
                n102 = property on="CAEN 1.2" class="Knob (strict)"("Scale.Minimum"="Scale.Range:Minimum 3", "Scale.Maximum"="Scale.Range:Maximum 3") -> ()  [unwired: 2 in, 2 out]
                n103 = property on="CAEN 1.3" class="Knob (strict)"("Scale.Maximum"="Scale.Range:Maximum 4", "Scale.Minimum"="Scale.Range:Minimum 4") -> ()  [unwired: 2 in, 2 out]
              }
              frame #2 {
                n104 = property on="CAEN 2.1" class="Knob (strict)"("Scale.Maximum"="Scale.Range:Maximum 6", "Scale.Minimum"="Scale.Range:Minimum 6") -> ()  [unwired: 2 in, 2 out]
                n105 = property on="CAEN 2.0" class="Knob (strict)"("Scale.Maximum"="Scale.Range:Maximum 5", "Scale.Minimum"="Scale.Range:Minimum 5") -> ()  [unwired: 2 in, 2 out]
              }
              frame #3 {
                n106 = property on="CAEN 2.2" class="Knob (strict)"("Scale.Maximum"="Scale.Range:Maximum 7", "Scale.Minimum"="Scale.Range:Minimum 7") -> ()  [unwired: 2 in, 2 out]
                n107 = property on="CAEN 2.3" class="Knob (strict)"("Scale.Maximum"="Scale.Range:Maximum 8", "Scale.Minimum"="Scale.Range:Minimum 8") -> ()  [unwired: 2 in, 2 out]
              }
            }
          }
          frame #1 {
            # "DAQmx Read above will replace dummy data below,\nonce the 9216 modules are functioning"
            # "Descr"
            # "NI 9207 8x V, 8x mA"
            # "Case to ignore runtime errors; unpack later"
            # "Module 1 tasks+status"
            # "Temps (NI)"
            # "9216 T     (NI) x16\n9207 V     (NI)  x8\n9207 mA (NI)  x8\nTemp        (LS)  x2\nHeater %           x1"
            # "Temp A, Temp B, heater power"
            # "Measurements and conversions"
            n108 = case shown="True" "Run lakeshore?" {
              tunnel: [w457 w468] -> w434
              tunnel: w433 -> [w457 w467]
              tunnel: [-273.0 ("Input A") w466] -> w430
              tunnel: [-273.0 ("Input B") w465] -> w429
              tunnel: [73.0 ("Heater 1 (%)") w464] -> w428
              tunnel: w427 -> [_ w462]
              tunnel: [-274.0 "Setpoint (°C)"] -> w424
              frame False {
              }
              frame True {
                # "LS output"
                # "P\nI\nD"
                n109 = Select(t=0, s=w462, f="Heater range") -> (s? t:f=w459:i32)
                n110 = Unbundle("PID settings") -> ("P"=w473:dbl, "I"=w472:dbl, "D"=w471:dbl)
                n111 = Unbundle(w467) -> ("VISA resource name out"=w475:refnum<visa-resource-name>, "error out"=w474:errorcluster)
                n112 = call "Lakeshore subVI.vi"("Setpoint"="Setpoint (°C)", "Rate (D) (X.X %)"=w471, "Range"=w459, "Reset (I) (XX.X)"=w472, "Gain (P) (XX.X)"=w473, "error in (no error)"=w474, "VISA resource name"=w475) -> ("Input B"=w465:dbl, "Input A"=w466:dbl, "error out"=w469:errorcluster, "VISA resource name out"=w470:refnum<visa-resource-name>, "Heater 1 (%)"=w464:dbl)
                "Lakeshore" <- w469
                n113 = Bundle("VISA resource name out"=w470, "error out"=w469) -> (w468:T5)  [unwired: 1 in]
              }
            }
            n114 = Get Date/Time In Seconds() -> (seconds since 1Jan1904=w432:timestamp)
            n115 = Quotient & Remainder(x=w420, y="Read T every N cycles") -> (x-y*floor(x/y)=w423:i32)  [unwired: 1 out]
            n116 = Unbundle(w405) -> ("task out"=w404:refnum<k21>, "error out"=w403:errorcluster)
            n117 = Build Array (concatenate)(w398, w432) -> (w431:timestamp[])
            n118 = Unbundle(w426) -> ("task out"=w410:refnum<k21>, "error out"=w409:errorcluster)
            n119 = case shown="1, Default" w423 {
              tunnel: w421 -> [_ w450]
              tunnel: [w443 w446] -> w418
              tunnel: w420 -> [w442 _]
              frame 0 {
                # "Dummy data"
                # "New temperatures"
                n120 = Add(x=w442, y=-95.0 ("element")) -> (x+y=w445:dbl)
                n121 = Initialize Array(w445, 16) -> (w443:dbl[])
              }
              frame 1, Default {
                # "Gets 1st 16 Col's\nfrom last row:\nPrevious 16 temps."
                # "Get previous temps"
                n122 = Array Size(array=w450) -> (size(s)=w452:i32[])
                n123 = Index Array(array=w452, index=0) -> (element=w453:i32)
                n124 = Decrement(x=w453) -> (x-1=w449:i32)
                n125 = Index Array(array=w450, index (row)=w449) -> (element=w448:dbl[])  [unwired: 1 in]
                n126 = Array Subset(array=w448, length=16) -> (w446:dbl[])  [unwired: 1 in]
              }
            }
            n127 = call-poly <vilib>:"DAQmx Read.vi"("task/channels in"=w404, "error in"=w403) -> ("task out"=w402:refnum<k21>, "data"=→"PT100 data":dbl[], "error out"=w401:errorcluster)  [unwired: 11 in]
            "NI 9216 x2" <- w401
            n128 = call-poly <vilib>:"DAQmx Read.vi"("task/channels in"=w410, "error in"=w409) -> ("task out"=w408:refnum<k21>, "data"=w417:dbl[], "error out"=w407:errorcluster)  [unwired: 11 in]
            "Raw readouts (V, mA)" <- w417
            "NI 9207" <- w407
            n129 = Build Array (concatenate)("Offsets\nsubtracted", "Offsets\nsubtracted") -> (w411:dbl[])
            n130 = Build Array (concatenate)("Multipliers", "Multipliers") -> (w414:dbl[])
            n131 = for {
              tunnel: w411 -> [w440] mode=indexing
              tunnel: w417 -> [w439] mode=indexing
              tunnel: w414 -> [w437] mode=indexing
              tunnel: [w436] -> w419 mode=indexing
              n132 = Subtract(x=w439, y=w440) -> (x-y=w438:dbl)
              n133 = Multiply(x=w438, y=w437) -> (x*y=w436:dbl)
            }
            n134 = Bundle("task out"=w402, "error out"=w401) -> (w400:T4)  [unwired: 1 in]
            n135 = Bundle("task out"=w408, "error out"=w407) -> (w422:T4)  [unwired: 1 in]
            n136 = Build Array(w430, w429, w428) -> (w406:dbl[])
            "LakeShore readings" <- w406
            n137 = Unbundle(w397) -> ("task out"=w396:refnum<k21>, "error out"=w395:errorcluster)
            n138 = call-poly <vilib>:"DAQmx Read.vi"("task/channels in"=w396, "error in"=w395) -> ("task out"=w394:refnum<k21>, "data"=→"PT1000 data":dbl[], "error out"=w393:errorcluster)  [unwired: 11 in]
            "NI 9226" <- w393
            n139 = Bundle("task out"=w394, "error out"=w393) -> (w392:T4)  [unwired: 1 in]
          }
          frame #2 {
            # "Alter voltages if button clicked"
            # "2"
            # "1"
            # "Descr."
            # "Descr."
            # "VMON1  x4 \nVMON2  x4\nIMON1    x4\nIMON2    x4"
            # "Needle gauge Voltage displays"
            # "1"
            # "2"
            # "1"
            # "2"
            # "Reads new V and A every N cycles,\nor passes previous values"
            # "High Voltage"
            n140 = Quotient & Remainder(x=w515, y="Read CAEN units \nevery N cycles") -> (x-y*floor(x/y)=w494:i32)  [unwired: 1 out]
            n141 = Unbundle(w522) -> ("VISA resource name out"=w482:refnum<visa-resource-name>, "error out"=w521:errorcluster)
            n142 = Unbundle(w519) -> ("VISA resource name out"=w481:refnum<visa-resource-name>, "error out"=w518:errorcluster)
            n143 = Build Array (concatenate)("VSet (V)", "VMax (V)", "IMax (uA)") -> (w499:dbl[])
            n144 = case shown="1, Default" w494 {
              tunnel: w482 -> [w673 _]
              tunnel: w521 -> [w672 w681]
              tunnel: w520 -> [_ w677]
              tunnel: w481 -> [w663 _]
              tunnel: w518 -> [w660 w682]
              tunnel: [w659 w682] -> w479
              tunnel: [w669 w681] -> w480
              tunnel: [w668 w677] -> w490
              tunnel: [w666 w678] -> w517
              tunnel: [w664 w674] -> w516
              frame 0 {
                # "All data x16"
                # "Voltages x8"
                # "Currents x8"
                # "Read"
                n145 = call "READ_SUPPLY.vi"("VISA resource name"=w673, "Board address"=u8 0, "NChannels"=u8 4, "error in (no error)"=w672) -> ("VMon values (V)"=w667:dbl[], "IMon values (uA)"=w665:dbl[], "error out"=w669:errorcluster)  [unwired: 9 in]
                n146 = call "READ_SUPPLY.vi"("VISA resource name"=w663, "Board address"=u8 0, "NChannels"=u8 4, "error in (no error)"=w660) -> ("VMon values (V)"=w658:dbl[], "IMon values (uA)"=w657:dbl[], "error out"=w659:errorcluster)  [unwired: 9 in]
                n147 = Build Array (concatenate)(w665, w657) -> (w664:dbl[])
                n148 = Build Array (concatenate)(w667, w658) -> (w666:dbl[])
                n149 = Build Array (concatenate)(w667, w658, w665, w657) -> (w668:dbl[])
              }
              frame 1, Default {
                # "Don't read: pass previous"
                n150 = Array Subset(array=w677, index=0, length=8) -> (w678:dbl[])
                n151 = Array Subset(array=w677, index=8, length=8) -> (w674:dbl[])
              }
            }
            "Voltages" <- w517
            "Vmon (V)" <- w517
            "IMon (uA)" <- w516
            n152 = Build Array("Apply Voltage", "Set to zero", "Kill voltage") -> (w493:bool[])
            n153 = case shown="True" "Query HV status" {
              tunnel: w482 -> [_ w534]
              tunnel: w481 -> [_ w533]
              tunnel: w479 -> [w523 w528]
              tunnel: w480 -> [w524 w527]
              tunnel: [w524 w526] -> w478
              tunnel: [w523 w525] -> w477
              frame False {
              }
              frame True {
                w536 = u8 0 ("Board address")
                w535 = u8 4 ("NChannels")
                n154 = Bundle("VISA resource name out"=w534, "Board address"=w536, "NChannels"=w535) -> (w531:T6)  [unwired: 1 in]
                n155 = Bundle("VISA resource name out"=w533, "Board address"=w536, "NChannels"=w535) -> (w532:T6)  [unwired: 1 in]
                n156 = call <instrlib>:"Channel Status.vi"("error in (no error)"=w527, "BoardHandle"=w531) -> ("error out"=w526:errorcluster, "Channel Status Array"=→"CAEN 1":T2)  [unwired: 7 in, 1 out]
                n157 = call <instrlib>:"Channel Status.vi"("error in (no error)"=w528, "BoardHandle"=w532) -> ("error out"=w525:errorcluster, "Channel Status Array"=→"CAEN 2":T2)  [unwired: 7 in, 1 out]
              }
            }
            n158 = Search 1D Array(1D array=w493, element=TRUE) -> (index of element=w507:i32)  [unwired: 1 in]
            n159 = case shown="1" w507 {
              tunnel: w482 -> [w562 w597 w630 w656]
              tunnel: w481 -> [w552 w589 w621 w655]
              tunnel: [w563 w598 w631 w654] -> w488
              tunnel: [w562 w597 w630 w656] -> w506
              tunnel: [w551 w588 w620 w653] -> w485
              tunnel: [w552 w589 w621 w655] -> w504
              tunnel: "VSet (V)" -> [w560 _ w628 _]
              tunnel: "VMax (V)" -> [w559 w595 _ _]
              tunnel: "IMax (uA)" -> [w558 w594 w627 _]
              tunnel: w478 -> [w550 w587 w619 w654]
              tunnel: w477 -> [w549 w586 w618 w653]
              frame 0 {
                w553 = 4 ("length")
                w557 = 4 ("length")
                # "Last four"
                # "First four"
                # "Apply voltage"
                n160 = Array Subset(array=w560, length=w557) -> (w565:dbl[])  [unwired: 1 in]
                n161 = Array Subset(array=w559, length=w557) -> (w564:dbl[])  [unwired: 1 in]
                n162 = Array Subset(array=w558, length=w557) -> (w561:dbl[])  [unwired: 1 in]
                n163 = Array Subset(array=w560, index=w553) -> (w556:dbl[])  [unwired: 1 in]
                n164 = Array Subset(array=w559, index=w553) -> (w555:dbl[])  [unwired: 1 in]
                n165 = Array Subset(array=w558, index=w553) -> (w554:dbl[])  [unwired: 1 in]
                n166 = for {
                  tunnel: w562 -> [w584]
                  tunnel: w550 -> [w583]
                  tunnel: w565 -> [w580] mode=indexing
                  tunnel: w564 -> [w578] mode=indexing
                  tunnel: w561 -> [w577] mode=indexing
                  tunnel: [w576] -> w563
                  i -> [w585]
                  n167 = call "SET_SUPPLY_CHANNEL.vi"("VISA resource name"=w584, "Voltage Level (0.0 V)"=w580, "Enable (OFF)"=TRUE, "Board address"=u8 0, "NChannels"=u8 4, "Channel (0)"=w585, "error in (no error)"=w583, "Voltage Max (0.0 V)"=w578, "Current Limit (0.00 uA)"=w577) -> ("error out"=w576:errorcluster)  [unwired: 6 in]
                }
                n168 = for {
                  tunnel: w552 -> [w575]
                  tunnel: w549 -> [w569]
                  tunnel: w556 -> [w574] mode=indexing
                  tunnel: w555 -> [w573] mode=indexing
                  tunnel: w554 -> [w572] mode=indexing
                  tunnel: [w568] -> w551
                  i -> [w571]
                  n169 = call "SET_SUPPLY_CHANNEL.vi"("VISA resource name"=w575, "Voltage Level (0.0 V)"=w574, "Enable (OFF)"=TRUE, "Board address"=u8 0, "NChannels"=u8 4, "Channel (0)"=w571, "error in (no error)"=w569, "Voltage Max (0.0 V)"=w573, "Current Limit (0.00 uA)"=w572) -> ("error out"=w568:errorcluster)  [unwired: 6 in]
                }
              }
              frame 1 {
                w590 = 4 ("length")
                w593 = 4 ("length")
                # "Set V to zero"
                n170 = Array Subset(array=w594, length=w593) -> (w596:dbl[])  [unwired: 1 in]
                n171 = Array Subset(array=w595, length=w593) -> (w599:dbl[])  [unwired: 1 in]
                n172 = Array Subset(array=w595, index=w590) -> (w592:dbl[])  [unwired: 1 in]
                n173 = Array Subset(array=w594, index=w590) -> (w591:dbl[])  [unwired: 1 in]
                n174 = for {
                  tunnel: w597 -> [w616]
                  tunnel: w587 -> [w615]
                  tunnel: w599 -> [w612] mode=indexing
                  tunnel: w596 -> [w611] mode=indexing
                  tunnel: [w610] -> w598
                  i -> [w617]
                  w609 = u8 0 ("Board address")
                  n175 = call "SET_SUPPLY_CHANNEL.vi"("VISA resource name"=w616, "Voltage Level (0.0 V)"=w609, "Enable (OFF)"=TRUE, "Board address"=w609, "NChannels"=u8 4, "Channel (0)"=w617, "error in (no error)"=w615, "Voltage Max (0.0 V)"=w612, "Current Limit (0.00 uA)"=w611) -> ("error out"=w610:errorcluster)  [unwired: 6 in]
                }
                n176 = for {
                  tunnel: w589 -> [w600]
                  tunnel: w586 -> [w605]
                  tunnel: w592 -> [w604] mode=indexing
                  tunnel: w591 -> [w603] mode=indexing
                  tunnel: [w601] -> w588
                  i -> [w606]
                  w608 = 0 ("length")
                  n177 = call "SET_SUPPLY_CHANNEL.vi"("VISA resource name"=w600, "Voltage Level (0.0 V)"=w608, "Enable (OFF)"=TRUE, "Board address"=w608, "NChannels"=u8 4, "Channel (0)"=w606, "error in (no error)"=w605, "Voltage Max (0.0 V)"=w604, "Current Limit (0.00 uA)"=w603) -> ("error out"=w601:errorcluster)  [unwired: 6 in]
                }
              }
              frame 2 {
                w622 = 4 ("length")
                w625 = 2 ("length")
                w626 = 4 ("length")
                # "CAEN 2: Top gate, Bottom gate"
                # "CAEN 1 values:\nPMT1&2, Anode, Cathode"
                # "Set VMax to zero, \"Kill\""
                n178 = Array Subset(array=w627, length=w626) -> (w629:dbl[])  [unwired: 1 in]
                n179 = Array Subset(array=w628, length=w626) -> (w632:dbl[])  [unwired: 1 in]
                n180 = Array Subset(array=w628, index=w622, length=w625) -> (w624:dbl[])
                n181 = Array Subset(array=w627, index=w622, length=w625) -> (w623:dbl[])
                n182 = for {
                  tunnel: w630 -> [w651]
                  tunnel: w619 -> [w650]
                  tunnel: w632 -> [w647] mode=indexing
                  tunnel: w629 -> [w645] mode=indexing
                  tunnel: [w644] -> w631
                  i -> [w652]
                  n183 = call "SET_SUPPLY_CHANNEL.vi"("VISA resource name"=w651, "Voltage Level (0.0 V)"=w647, "Enable (OFF)"=TRUE, "Board address"=u8 0, "NChannels"=u8 4, "Channel (0)"=w652, "error in (no error)"=w650, "Voltage Max (0.0 V)"=u8 0 ("Board address"), "Current Limit (0.00 uA)"=w645) -> ("error out"=w644:errorcluster)  [unwired: 6 in]
                }
                n184 = for {
                  tunnel: w621 -> [w633]
                  tunnel: w618 -> [w636]
                  tunnel: w624 -> [w639] mode=indexing
                  tunnel: w623 -> [w637] mode=indexing
                  tunnel: [w635] -> w620
                  i -> [w642]
                  n185 = call "SET_SUPPLY_CHANNEL.vi"("VISA resource name"=w633, "Voltage Level (0.0 V)"=w639, "Enable (OFF)"=TRUE, "Board address"=u8 0, "NChannels"=u8 4, "Channel (0)"=w642, "error in (no error)"=w636, "Voltage Max (0.0 V)"=0, "Current Limit (0.00 uA)"=w637) -> ("error out"=w635:errorcluster)  [unwired: 6 in]
                }
              }
              frame 3, Default {
                # "\"Executes\" if none of the three buttons have been clicked"
                # "Do nothing"
              }
            }
            n186 = Unbundle(w480) -> ("status"=w489:bool)  [unwired: 2 out]
            n187 = Unbundle(w479) -> ("status"=w486:bool)  [unwired: 2 out]
            n188 = stacked-sequence {
              tunnel: w489 -> [w540 _]
              tunnel: w480 -> [w538 _]
              tunnel: w488 -> [w539 _]
              tunnel: [w537 _] -> w487
              tunnel: w486 -> [_ w543]
              tunnel: w479 -> [_ w546]
              tunnel: w485 -> [_ w545]
              tunnel: [_ w544] -> w484
              frame #0 {
                n189 = case shown="False" w540 {
                  tunnel: w539 -> [w541 _]
                  tunnel: w538 -> [_ w542]
                  tunnel: [w541 w542] -> w537
                  frame False {
                  }
                  frame True {
                  }
                }
              }
              frame #1 {
                n190 = case shown="False" w543 {
                  tunnel: w546 -> [_ w548]
                  tunnel: w545 -> [w547 _]
                  tunnel: [w547 w548] -> w544
                  frame False {
                  }
                  frame True {
                  }
                }
              }
            }
            "CAEN 1" <- w487
            "CAEN 2" <- w484
            n191 = Bundle("VISA resource name out"=w506, "error out"=w488) -> (w505:T5)  [unwired: 1 in]
            n192 = Bundle("VISA resource name out"=w504, "error out"=w485) -> (w503:T5)  [unwired: 1 in]
            n193 = Index Array(array=w490) -> (element #1=→"CAEN 1.0":dbl, element #2=→"CAEN 1.1":dbl, element #3=→"CAEN 1.2":dbl, element #4=→"CAEN 1.3":dbl, element #5=→"CAEN 2.0":dbl, element #6=→"CAEN 2.1":dbl, element #7=→"CAEN 2.2":dbl, element #8=→"CAEN 2.3":dbl)  [unwired: 8 in]
          }
          frame #3 {
            # "Descr."
            # "Reset anode"
            n194 = Or Array Elements(Boolean array=w684) -> (logical OR=w683:bool)
            n195 = case shown="True" "Reset anode\nperiodically?" {
              tunnel: w691 -> [_ w697]
              tunnel: w690 -> [_ w706]
              tunnel: w689 -> [_ w711]
              tunnel: w683 -> [_ w695]
              tunnel: [w692 w696] -> w686
              tunnel: w685 -> [_ w705]
              frame False {
                # "Anode Reset Routine inactive:\nkeep timers up to date so activating\nroutine will correctly initiate the timers."
                n196 = Get Date/Time In Seconds() -> (seconds since 1Jan1904=w694:timestamp)
                n197 = To Double Precision Float(number=w694) -> (double precision float=w693:dbl)
                n198 = Build Array(w693, w693) -> (w692:dbl[])
              }
              frame True {
                # "Descr."
                n199 = case shown="\"CAEN 1\", Default" "CAEN unit selector" {
                  tunnel: w706 -> [w725 _]
                  tunnel: w705 -> [_ w727]
                  tunnel: [w725 w727] -> w704
                  tunnel: [0 4] -> w702
                  frame "CAEN 1", Default {
                  }
                  frame "CAEN 2" {
                  }
                }
                n200 = call "anode_timing.vi"("Keep off for X seconds"="Keep off for X seconds", "Array of timers"=w697, "Kill every Y minutes"="Kill every Y minutes") -> ("Time to kill"=w713:bool, "Time until reset"=→"Seconds until \nanode reset":dbl, "Time until autokill"=→"Seconds until \nanode autokill":dbl, "Time to reset"=w714:bool)  [unwired: 5 in]
                "Killed" <- w713
                "Restarted" <- w714
                n201 = Add(x=w702, y="Anode ch.") -> (x+y=w700:i32)
                n202 = Build Array(w713, w714, w695) -> (w717:bool[])
                n203 = Add(x=w700, y=8) -> (x+y=w707:i32)
                n204 = Add(x=w700, y=16) -> (x+y=w708:i32)
                n205 = Search 1D Array(1D array=w717, element=TRUE) -> (index of element=w716:i32)  [unwired: 1 in]
                n206 = Unbundle(w704) -> ("VISA resource name out"=w722:refnum<visa-resource-name>, "error out"=w721:errorcluster)
                n207 = Index Array(array=w711, index #1=w700, index #2=w707, index #3=w708) -> (element #1=w720:dbl, element #2=w718:dbl, element #3=w719:dbl)
                n208 = case shown="2" w716 {
                  tunnel: w720 -> [_ w751 _ _]
                  tunnel: w718 -> [w736 w750 _ _]
                  tunnel: w719 -> [w738 w749 _ _]
                  tunnel: w722 -> [w743 w754 _ _]
                  tunnel: w721 -> [w742 w753 _ _]
                  tunnel: "Anode ch." -> [w734 w747 _ _]
                  tunnel: w697 -> [w729 _ _ w760]
                  tunnel: [w728 w744 w757 w760] -> w696
                  frame 0 {
                    # "Set Anode Voltage to zero,\nreset the 1st timer"
                    # "Anode Vset to zero"
                    n209 = Get Date/Time In Seconds() -> (seconds since 1Jan1904=w732:timestamp)
                    n210 = Index Array(array=w729, index=1) -> (element=w730:dbl)
                    n211 = To Double Precision Float(number=w732) -> (double precision float=w731:dbl)
                    n212 = call "SET_SUPPLY_CHANNEL.vi"("VISA resource name"=w743, "Voltage Level (0.0 V)"=0.0, "Enable (OFF)"=TRUE, "Board address"=u8 0, "NChannels"=u8 4, "Channel (0)"=w734, "error in (no error)"=w742, "Voltage Max (0.0 V)"=w736, "Current Limit (0.00 uA)"=w738) -> ("error out"=w737:errorcluster)  [unwired: 6 in]
                    n213 = Build Array(w731, w730) -> (w728:dbl[])
                    n214 = call <vilib>:"Simple Error Handler.vi"("error in (no error)"=w737) -> ()  [unwired: 4 in, 5 out]
                  }
                  frame 1 {
                    # "Set Anode Voltage to defined value,\nreset both timers"
                    # "Anode Vset applied"
                    n215 = Get Date/Time In Seconds() -> (seconds since 1Jan1904=w746:timestamp)
                    n216 = To Double Precision Float(number=w746) -> (double precision float=w745:dbl)
                    n217 = call "SET_SUPPLY_CHANNEL.vi"("VISA resource name"=w754, "Voltage Level (0.0 V)"=w751, "Enable (OFF)"=TRUE, "Board address"=u8 0, "NChannels"=u8 4, "Channel (0)"=w747, "error in (no error)"=w753, "Voltage Max (0.0 V)"=w750, "Current Limit (0.00 uA)"=w749) -> ("error out"=w748:errorcluster)  [unwired: 6 in]
                    n218 = Build Array(w745, w745) -> (w744:dbl[])
                    n219 = call <vilib>:"Simple Error Handler.vi"("error in (no error)"=w748) -> ()  [unwired: 4 in, 5 out]
                  }
                  frame 2 {
                    # "Change Voltage button pressed"
                    # "Reset both timers"
                    n220 = Get Date/Time In Seconds() -> (seconds since 1Jan1904=w759:timestamp)
                    n221 = To Double Precision Float(number=w759) -> (double precision float=w758:dbl)
                    n222 = Build Array(w758, w758) -> (w757:dbl[])
                  }
                  frame 3, Default {
                    # "Timers stay at previous value,\nso difference between those and\ncurrent time keeps incrementing"
                    # "No event"
                  }
                }
              }
            }
            n223 = To Time Stamp(1:w686) -> (0:→"Anode timers":timestamp[])
            "?" <- "Reset anode\nperiodically?"
          }
          frame #4 {
            w779 = 16 ("index")
            # "Plots 9207 output vs time"
            # "Descr."
            # "Moving averages"
            # "Historic graphs: Phase, 9207 ai, Flow, Heater, Temperature"
            # "Non-historic Temperature + Det. Pressure"
            # "Updated TOBA"
            # "Descr."
            # "Latest Detector Pressure"
            # "Plots individual lists of Temp. vs. t"
            # "Plots and moving averages"
            n224 = Build Array (concatenate)(w790, w799, w797) -> (w798:dbl[])
            n225 = Build Array (concatenate)(w800, w798) -> (w777:dbl[][])
            "TOBA appended" <- w777
            n226 = local read "Det. T."() -> (w771:i32[])
            n227 = local read "Flow input #"() -> (w767:i32)
            n228 = local read "Det.P input #"() -> (w768:i32)
            n229 = Equal?(x=666, y="Temperature channel selector") -> (x = y?=w791:bool)
            n230 = case shown="True" w791 {
              tunnel: w790 -> [w833 w839]
              tunnel: w771 -> [_ w838]
              tunnel: [w832 w834] -> w788
              tunnel: "Temperature channel selector" -> [w831 _]
              frame False {
                n231 = Index Array(array=w833, index=w831) -> (element=w832:dbl)
              }
              frame True {
                n232 = for {
                  tunnel: w839 -> [w842]
                  tunnel: w838 -> [w841] mode=indexing
                  tunnel: [w840] -> w835 mode=indexing
                  n233 = Index Array(array=w842, index=w841) -> (element=w840:dbl)
                }
                n234 = Array Size(array=w835) -> (size(s)=w837:i32)
                n235 = Add Array Elements(numeric array=w835) -> (sum=w836:dbl)
                n236 = Divide(x=w836, y=w837) -> (x/y=w834:dbl)
              }
            }
            n237 = Add(x=w768, y=w779) -> (x+y=w781:i32)
            n238 = Add(x=w779, y=w767) -> (x+y=w778:i32)
            n239 = Index Array(array=w777, index (col)=34 ("disabled index (col)")) -> (element=w784:dbl[])  [unwired: 1 in]
            n240 = Index Array(array=w777, index (col) #1=w781, index (col) #2=w778) -> (element #1=w780:dbl[], element #2=w765:dbl[])  [unwired: 2 in]
            n241 = Index Array(array=w777, index (col)="Temperature Channel Selector") -> (element=w786:dbl[])  [unwired: 1 in]
            n242 = local read "Det.P input #"() -> (w769:i32)
            n243 = Bundle(w786, w780) -> (w806:cluster{dbl[], dbl[]})  [unwired: 1 in]
            n244 = for {
              N: 8 -> [_]
              tunnel: w777 -> [w823]
              tunnel: w761 -> [w815]
              tunnel: [w820] -> w775 mode=indexing
              tunnel: [w814] -> w774 mode=indexing
              i -> [w819]
              n245 = Add(x=w819, y=24) -> (x+y=w817:i32)
              n246 = Add(x=16, y=w819) -> (x+y=w822:i32)
              n247 = Index Array(array=w823, index (col) #1=w822, index (col) #2=w817) -> (element #1=w821:dbl[], element #2=w816:dbl[])  [unwired: 2 in]
              n248 = Bundle(w815, w821) -> (w820:cluster{timestamp[], dbl[]})  [unwired: 1 in]
              n249 = Bundle(w815, w816) -> (w814:cluster{timestamp[], dbl[]})  [unwired: 1 in]
            }
            "9207 (ai 0:7, Volts)" <- w775
            "9207 (ai 8:15, Amperes)" <- w774
            n250 = Bundle(w761, w765) -> (w804:cluster{timestamp[], dbl[]})  [unwired: 1 in]
            n251 = Build Array(w804) -> (→"Flow (SLPM)":cluster{timestamp[], dbl[]}[])
            n252 = Index Array(array=w799, index=w769) -> (element=w807:dbl)
            n253 = Build Array(w806) -> (→"Historical Large Phase Diagram":cluster{dbl[], dbl[]}[])
            n254 = Bundle(w788, w807) -> (w811:cluster{dbl, dbl})  [unwired: 1 in]
            n255 = Bundle(w761, w784) -> (w802:cluster{timestamp[], dbl[]})  [unwired: 1 in]
            n256 = Build Array(w811) -> (→"Phase Diagram":cluster{dbl, dbl}[])
            n257 = Build Array(w802) -> (→"Heater power (%)":cluster{timestamp[], dbl[]}[])
            n258 = local read "Det. T."() -> (w770:i32[])
            n259 = Equal?(x=666, y="Temperature Channel Selector") -> (x = y?=w793:bool)
            n260 = call "moving_avg.vi"("N samples"="N samples", "Array"=w780) -> ("Numeric"=→"Detector Pressure":dbl)  [unwired: 9 in]
            n261 = call "moving_avg.vi"("N samples"="N samples", "Array"=w765) -> ("Numeric"=→"Average Flow (SLPM)":dbl)  [unwired: 9 in]
            n262 = for {
              N: 16 -> [_]
              tunnel: w761 -> [w859]
              tunnel: [w858] -> w812 mode=indexing
              tunnel: w777 -> [w857]
              i -> [w856]
              n263 = Index Array(array=w857, index (col)=w856) -> (element=w855:dbl[])  [unwired: 1 in]
              n264 = Bundle(w859, w855) -> (w858:cluster{timestamp[], dbl[]})  [unwired: 1 in]
            }
            "Temperature (ai 0:15, °C)" <- w812
            n265 = case shown="True" w793 {
              tunnel: w790 -> [w845 w851]
              tunnel: w770 -> [_ w850]
              tunnel: [w844 w846] -> w796
              tunnel: "Temperature Channel Selector" -> [w843 _]
              frame False {
                n266 = Index Array(array=w845, index=w843) -> (element=w844:dbl)
              }
              frame True {
                n267 = for {
                  tunnel: w851 -> [w854]
                  tunnel: w850 -> [w853] mode=indexing
                  tunnel: [w852] -> w847 mode=indexing
                  n268 = Index Array(array=w854, index=w853) -> (element=w852:dbl)
                }
                n269 = Array Size(array=w847) -> (size(s)=w849:i32)
                n270 = Add Array Elements(numeric array=w847) -> (sum=w848:dbl)
                n271 = Divide(x=w848, y=w849) -> (x/y=w846:dbl)
              }
            }
            n272 = local read "Channel Names (9207, ai8:15)"() -> (w773:string[])
            n273 = local read "Channel Names (9207, ai0:7)"() -> (w772:string[])
            n274 = call "Is Value Changed.vim"("value"=w773) -> ("changed or first call?"=w782:bool)
            n275 = call "Is Value Changed.vim"("value"=w772) -> ("changed or first call?"=w783:bool)
            n276 = Bundle(w796, w807) -> (w809:cluster{dbl, dbl})  [unwired: 1 in]
            n277 = case shown="True" w782 {
              tunnel: w773 -> [_ w825]
              frame False {
              }
              frame True {
                n278 = for {
                  tunnel: w825 -> [w826] mode=indexing
                  i -> [w827]
                  n279 = property on="9207 (ai 8:15, Amperes)" class="XYGraph (strict)"("Active Plot"=w827, "Plot.Plot Name"=w826) -> ()  [unwired: 2 in, 2 out]
                }
              }
            }
            n280 = case shown="True" w783 {
              tunnel: w772 -> [_ w828]
              frame False {
              }
              frame True {
                n281 = for {
                  tunnel: w828 -> [w829] mode=indexing
                  i -> [w830]
                  n282 = property on="9207 (ai 0:7, Volts)" class="XYGraph (strict)"("Active Plot"=w830, "Plot.Plot Name"=w829) -> ()  [unwired: 2 in, 2 out]
                }
              }
            }
            n283 = Build Array(w809) -> (→"Large Phase Diagram":cluster{dbl, dbl}[])
          }
          frame #5 {
            # "Temp A, Temp B, Heater%"
            # "Temperatures x16\nTo indicators on the physical schematic"
            # "Individual latest 9207 readings.\nIndicators go here. Array is 1x16,\nitems have been converted using\nthe offsets and multipliers"
            # "Displays"
            n284 = local read "Flow input #"() -> (w863:i32)
            n285 = case shown="False" "Reset?" {
              tunnel: [w875 0.0] -> w871
              tunnel: w868 -> [w875 _]
              frame False {
              }
              frame True {
              }
            }
            n286 = Index Array(array=w862) -> ()  [unwired: 16 in, 16 out]
            n287 = Index Array(array=w862, index=w863) -> (element=w866:dbl)
            n288 = call "Average_flow_x_time.vi"("Array of timestamps"=w870, "Previous Flow"=w869, "Latest Flow"=w866) -> ("Volume (SL)"=w872:dbl)  [unwired: 8 in]
            n289 = case shown="False" "Pause?" {
              tunnel: w871 -> [w879 w880]
              tunnel: w872 -> [w878 _]
              tunnel: [w877 w880] -> w867
              frame False {
                n290 = Add(x=w878, y=w879) -> (x+y=w877:dbl)
              }
              frame True {
              }
            }
            "Integrated Flow (SL)" <- w867
            n291 = Index Array(array=w864) -> (element #1=→"Coldhead" →"Temp A":dbl, element #2=→"Heater" →"Temp B":dbl)  [unwired: 3 in, 1 out]
            n292 = Index Array(array=w865) -> ()  [unwired: 16 in, 16 out]
            "9207 (V; A) Converted" <- w862
            "9216 #1 (°C)" <- w865
            "9216 #2 (°C)" <- w865
          }
          frame #6 {
            # "The same order applies to the headers re-saved,\nbut with an additional line, stating the date/time"
            # "-----------DATA SAVED----------\nHuman-readable timestamp  ;\nTemperatures (16),  2xNI 9216;\nVolts, Amps  (8 x2),     NI 9207;\nTemperature (2),    Lakeshore;\nHeater power (1),  Lakeshore;\nSetpoint (1),           Lakeshore;\nHV readouts (16)          CAEN ;\nCurrent time (s)                ---   ;\nCycle time (s)                    ---   ;"
            # "Saving data"
            n293 = Get Date/Time In Seconds() -> (seconds since 1Jan1904=w898:timestamp)
            n294 = To Double Precision Float(number=w898) -> (double precision float=w883:dbl)
            n295 = Build Array (concatenate)(w887, w886, w885, w899, w884, w883, w882) -> (w897:dbl[])
            n296 = Get Date/Time String() -> (date string=w891:string)  [unwired: 3 in, 1 out]
            n297 = case shown="True" "Re-save headers" {
              frame False {
                # "Just sit around and feel pretty"
              }
              frame True {
                w907 = ""
                # "Append line of most recent channel names to header file"
                n298 = local read "Channel Names (CAEN)"() -> (w906:string[])
                n299 = local read "Channel Names (9207, ai0:7)"() -> (w914:string[])
                n300 = for {
                  N: 16 -> [_]
                  shift-right: [w939] -> w910
                  shift-left: "" -> [w940]
                  i -> [w944]
                  n301 = Format Into String(initial string="t", w944) -> (resulting string=w942:string)  [unwired: 2 in, 1 out]
                  n302 = Concatenate Strings(w940, w942, "\t") -> (w939:string)
                }
                n303 = for {
                  shift-right: [w937] -> w912
                  shift-left: w907 -> [w938]
                  tunnel: w914 -> [w935] mode=indexing
                  n304 = Concatenate Strings(w938, w935, "\t") -> (w937:string)
                }
                n305 = local read "Channel Names (9207, ai8:15)"() -> (w913:string[])
                n306 = for {
                  tunnel: w906 -> [w929] mode=indexing
                  shift-right: [w927] -> w901
                  shift-left: w907 -> [w926]
                  n307 = Concatenate Strings(w926, w929, " (V)", "\t") -> (w927:string)
                }
                n308 = for {
                  shift-right: [w933] -> w909
                  shift-left: w912 -> [w934]
                  tunnel: w913 -> [w931] mode=indexing
                  n309 = Concatenate Strings(w934, w931, "\t") -> (w933:string)
                }
                n310 = for {
                  tunnel: w906 -> [w924] mode=indexing
                  shift-right: [w922] -> w905
                  shift-left: w901 -> [w921]
                  n311 = Concatenate Strings(w921, w924, " (I)", "\t") -> (w922:string)
                }
                n312 = Get Date/Time String() -> (date string=w919:string)  [unwired: 3 in, 1 out]
                n313 = Format Date/Time String() -> (date/time string=w900:string)  [unwired: 3 in]
                n314 = Build Path(base path=path "D:/Log_data/SC_LOG_HEADERS", name or relative path=w919) -> (appended path=w918:path)
                n315 = Concatenate Strings("Time\t", w910, w909, "Temp A\tTemp B\tHeater Power\tSetpoint\t", w905, "Time in seconds\tTime per cycle\t", w900, "\r\n") -> (w902:string)
                n316 = call <vilib>:"Write Spreadsheet String.vi"("append to file? (new file:F)"=TRUE, "spreadsheet string"=w902, "file path (dialog if empty)"=w918) -> ()  [unwired: 7 in, 2 out]
              }
            }
            n317 = Build Path(base path=path "D:/Log_data/SC_LOG", name or relative path=w891) -> (appended path=w890:path)
            n318 = Format Date/Time String() -> (date/time string=w895:string)  [unwired: 3 in]
            n319 = Array To Spreadsheet String(array=w897, 3:"%.3f" ("format string")) -> (spreadsheet string=w893:string)  [unwired: 1 in]
            n320 = Concatenate Strings(w895, "\t", w893) -> (w889:string)
            n321 = call <vilib>:"Write Spreadsheet String.vi"("append to file? (new file:F)"=TRUE, "spreadsheet string"=w889, "file path (dialog if empty)"=w890) -> ()  [unwired: 7 in, 2 out]
          }
          frame #7 {
            # "Status is True if ANY (armed)\ncondition is met"
            # "Detector P. Alert"
            # "Uninteruptable\n Power Supply Alert"
            # "Temp. Warning"
            # "Arms"
            # "Comm. Alert"
            # "Temperature Alert"
            # "Alarm conditions (Temp)"
            # "Check Alarms and Warnings"
            n322 = Unbundle By Name(w989) -> ("error out.status"=w970:bool)
            "NI mod 2&3 status" <- w970
            n323 = Unbundle By Name(w1002) -> ("error out.status"=w1000:bool)
            "LakeShore status" <- w1000
            n324 = Unbundle By Name(w1004) -> ("error out.status"=w999:bool)
            "CAEN 1 status" <- w999
            n325 = Unbundle By Name(w1003) -> ("error out.status"=w998:bool)
            "CAEN 2 status" <- w998
            n326 = Unbundle By Name(w1001) -> ("error out.status"=w997:bool)
            "NI mod1 (P) status" <- w997
            n327 = Build Array(w1000, w999, w998, w997, w970) -> (w971:bool[])
            n328 = Build Array("LakeShore", "CAEN 1", "CAEN 2", "NI mod 2&3", "NI mod 1") -> (w966:bool[])
            n329 = call "check_ups.vi"() -> ("Error: no voltages read"=w950:bool, "Timestamp last measured"=→"Timestamp last \nmeasured (UPS)":timestamp, "Minimum input voltage measured"=w960:dbl)  [unwired: 8 in, 1 out]
            "Minimum input voltage measured" <- w960
            n330 = property on="Det.P input #" class="DigNum (strict)"() -> ("Value"=w986:i32)  [unwired: 2 in, 2 out]
            n331 = Or Array Elements(Boolean array=w971) -> (logical OR=→"Comm. status":bool)
            n332 = for {
              tunnel: w971 -> [w1007] mode=indexing
              tunnel: w966 -> [w1006] mode=indexing
              tunnel: [w1005] -> w965 mode=indexing
              n333 = And(x=w1007, y=w1006) -> (x .and. y?=w1005:bool)
            }
            n334 = Index Array(array=w987, index=w986) -> (element=w983:dbl)
            n335 = Less?(x=w960, y="UPS Voltage \nLower Threshold") -> (x < y?=w952:bool)
            n336 = Equal?(x=w960, y=-1.0) -> (x = y?=w951:bool)
            n337 = Less?(x=w983, y="Underpressure threshold") -> (x < y?=w981:bool)
            n338 = Build Array(w952, w951, w950) -> (w949:bool[])
            n339 = Or Array Elements(Boolean array=w965) -> (logical OR=w955:bool)
            n340 = Greater?(x=w983, y="Overpressure threshold") -> (0:w982:bool)
            n341 = Or(x=w982, y=w981) -> (x .or. y?=w980:bool)
            "Det. P. warning" <- w980
            n342 = Or Array Elements(Boolean array=w949) -> (logical OR=w948:bool)
            "Warning" <- w948
            n343 = And(x="UPS", y=w948) -> (x .and. y?=w954:bool)
            n344 = And(x=w980, y="Detector Pressure") -> (x .and. y?=w956:bool)
            n345 = local read "Det. T."() -> (w946:i32[])
            n346 = Build Array("T 1", "T 2", "T 3", "T 4", "T 5", "T 6") -> (w945:bool[])
            n347 = for {
              tunnel: w988 -> [w1017]
              tunnel: w946 -> [w1016] mode=indexing
              tunnel: w945 -> [w1010] mode=indexing
              tunnel: [w1009] -> w957 mode=indexing
              tunnel: [w1008] -> w972 mode=indexing
              n348 = Index Array(array=w1017, index=w1016) -> (element=w1013:dbl)
              n349 = Less?(x=w1013, y="Low Temp threshold") -> (x < y?=w1012:bool)
              n350 = Greater?(x=w1013, y="High Temp threshold") -> (0:w1011:bool)
              n351 = Or(x=w1012, y=w1011) -> (x .or. y?=w1008:bool)
              n352 = And(x=w1010, y=w1008) -> (x .and. y?=w1009:bool)
            }
            n353 = Index Array(array=w972) -> (element #1=→"Boolean":bool, element #2=→"Boolean 2":bool, element #3=→"Boolean 3":bool, element #4=→"Boolean 4":bool, element #5=→"Boolean 5":bool, element #6=→"Boolean 6":bool)  [unwired: 6 in]
            n354 = Build Array (concatenate)(w957, w956, w955, w954) -> (w953:bool[])
            n355 = Or Array Elements(Boolean array=w953) -> (logical OR=w947:bool)
            "Alarm state" <- w947
          }
          frame #8 {
            # "Testing alarm will not interfere"
            # "Act on alarm"
            n356 = Or(x="Test alarm", y=w1024) -> (x .or. y?=w1025:bool)
            n357 = case shown="True" w1025 {
              tunnel: "Test alarm" -> [_ w1032]
              tunnel: w1022 -> [_ w1040]
              tunnel: w1021 -> [_ w1039]
              tunnel: w1020 -> [w1028 w1030]
              tunnel: "Alarm\nMaster switch" -> [_ w1037]
              tunnel: [w1028 w1031] -> w1018
              frame False {
                # "Timer stays at previous value"
              }
              frame True {
                n358 = Get Date/Time In Seconds() -> (seconds since 1Jan1904=w1044:timestamp)
                n359 = case shown="True" "\"Sound\" alarm" {
                  frame False {
                  }
                  frame True {
                    n360 = call <vilib>:"Beep.vi"("duration (msec)"=u32 1000, "frequency (Hz)"="Sound alarm\nFrequency (Hz)") -> ()  [unwired: 10 in]
                  }
                }
                n361 = To Double Precision Float(number=w1044) -> (double precision float=w1041:dbl)
                n362 = Multiply(x="Repeat Alarm SMS\nevery N minutes", y=60.0) -> (x*y=w1033:dbl)
                n363 = Subtract(x=w1041, y=w1030) -> (x-y=w1036:dbl)
                n364 = Greater?(x=w1036, y=w1033) -> (0:w1038:bool)
                n365 = And(x=w1037, y=w1038) -> (x .and. y?=w1035:bool)
                n366 = Or(x=w1032, y=w1035) -> (x .or. y?=w1034:bool)
                n367 = case shown="True" w1034 {
                  tunnel: w1032 -> [_ w1059]
                  tunnel: w1040 -> [_ w1067]
                  tunnel: w1039 -> [_ w1055]
                  tunnel: [w1047 w1057] -> w1031
                  tunnel: w1030 -> [w1047 w1056]
                  frame False {
                    # "Alarm not armed, or defined time has not yet passed"
                  }
                  frame True {
                    # "Average T in Det."
                    n368 = local read "Det. T."() -> (w1073:i32[])
                    n369 = local read "Det.P input #"() -> (w1074:i32)
                    n370 = case shown="True" w1059 {
                      tunnel: ["Error encountered inXAMS! Status:" "TESTING the XAMS alarm. Status:"] -> w1066
                      tunnel: [w1078 w1081] -> w1057
                      tunnel: w1056 -> [_ w1081]
                      frame False {
                        n371 = Get Date/Time In Seconds() -> (seconds since 1Jan1904=w1079:timestamp)
                        n372 = To Double Precision Float(number=w1079) -> (double precision float=w1078:dbl)
                      }
                      frame True {
                      }
                    }
                    n373 = for {
                      tunnel: w1055 -> [w1092]
                      tunnel: w1073 -> [w1088] mode=indexing
                      tunnel: [w1091] -> w1072 mode=indexing
                      tunnel: [w1089] -> w1050 mode=indexing
                      n374 = Index Array(array=w1092, index=w1088) -> (element=w1091:dbl)
                      n375 = Format Into String(format string="%.0f", w1088) -> (resulting string=w1086:string)  [unwired: 2 in, 1 out]
                      n376 = Format Into String(format string="%.1f", w1091) -> (resulting string=w1084:string)  [unwired: 2 in, 1 out]
                      n377 = Concatenate Strings("\n" ("format string"), w1086, "     " ("format string"), w1084) -> (w1089:string)
                    }
                    n378 = Index Array(array=w1067, index=w1074) -> (element=w1068:dbl)
                    n379 = Array Size(array=w1072) -> (size(s)=w1070:i32)
                    n380 = Add Array Elements(numeric array=w1072) -> (sum=w1071:dbl)
                    n381 = Format Into String(format string="%.3f", w1068) -> (resulting string=w1062:string)  [unwired: 2 in, 1 out]
                    n382 = Divide(x=w1071, y=w1070) -> (x/y=w1060:dbl)
                    n383 = Format Date/Time String() -> (date/time string=w1064:string)  [unwired: 3 in]
                    n384 = Format Into String(format string="%.2f", w1060) -> (resulting string=w1048:string)  [unwired: 2 in, 1 out]
                    n385 = Concatenate Strings(w1066, "\nDate/time: ", w1064, "\nDetector Pressure: ", w1062, " bar", "\nDetector Temperatures (°C):", "\nCh:   Temp:" ("format string"), w1050, "\nAverage detector temperature: ", w1048) -> (w1054:string)
                    "Alarm (or test) message" <- w1054
                    n386 = for {
                      tunnel: w1054 -> [w1077]
                      tunnel: "Phone numbers" -> [w1076] mode=indexing
                      n387 = call "send_sms.vi"("Message content"=w1077, "Phone number"=w1076) -> ("standard error"=→"SMS error":string)  [unwired: 8 in, 1 out]
                    }
                  }
                }
              }
            }
            n388 = And(x="Shut off heater \nif Alarm is active", y=w1024) -> (x .and. y?=w1026:bool)
            "Alarm active 2" <- "Alarm\nMaster switch"
          }
          frame #9 {
            # "Daily e-mail"
            n389 = Get Date/Time In Seconds() -> (seconds since 1Jan1904=w1105:timestamp)
            n390 = To Double Precision Float(number=w1105) -> (double precision float=w1104:dbl)
            n391 = Get Date/Time String(want seconds? (F)=FALSE) -> (time string=w1107:string)  [unwired: 2 in, 1 out]
            n392 = Subtract(x=w1104, y=w1097) -> (x-y=w1103:dbl)
            n393 = Equal?(x=w1107, y="Send status email at time:") -> (x = y?=w1100:bool)
            n394 = Greater?(x=w1103, y=62) -> (0:w1099:bool)
            n395 = Build Array("Send daily email?", w1100, w1099) -> (w1098:bool[])
            n396 = And Array Elements(Boolean array=w1098) -> (logical AND=w1094:bool)
            n397 = Or(x="Send status email now", y=w1094) -> (x .or. y?=w1095:bool)
            n398 = case shown="True" w1095 {
              tunnel: w1111 -> [_ w1146]
              tunnel: w1110 -> [_ w1129]
              tunnel: w1109 -> [_ w1138]
              tunnel: w1097 -> [w1112 _]
              tunnel: [w1112 w1124] -> w1096
              frame False {
              }
              frame True {
                # "Average T in Det."
                n399 = local read "Det. T."() -> (w1147:i32[])
                n400 = Not Equal To 0?(x="Number of Bonus lines") -> (x != 0?=w1117:bool)
                n401 = case shown="True" w1117 {
                  tunnel: [w1152 w1155] -> w1118
                  tunnel: "Number of Bonus lines" -> [_ w1158]
                  frame False {
                    n402 = Build Array("\n[Flavor text module inactive]") -> (w1152:string[])
                  }
                  frame True {
                    n403 = Build Path(base path=path "C:/Users/xams/Desktop/New XAMS Slow Control", name or relative path="cool_beans.txt") -> (appended path=w1159:path)
                    n404 = call-poly <vilib>:"Read Delimited Spreadsheet.vi"("file path (dialog if empty)"=w1159) -> ("all rows"=w1162:string[][])  [unwired: 9 in, 5 out]
                    n405 = Array Size(array=w1162) -> (size(s)=w1164:i32[])
                    n406 = Index Array(array=w1164) -> (element=w1163:i32)  [unwired: 1 in]
                    n407 = for {
                      N: w1158 -> [_]
                      tunnel: w1163 -> [w1169]
                      tunnel: w1162 -> [w1168]
                      tunnel: [w1165] -> w1156 mode=indexing
                      n408 = Random Number (0-1)() -> (number: 0 to 1=w1172:dbl)
                      n409 = Multiply(x=w1169, y=w1172) -> (x*y=w1171:dbl)
                      n410 = Round To Nearest(number=w1171) -> (nearest integer value=w1170:dbl)
                      n411 = Index Array(array=w1168, index (row)=w1170) -> (element=w1166:string[])  [unwired: 1 in]
                      n412 = Concatenate Strings("\n", w1166) -> (w1165:string)
                    }
                    n413 = Concatenate Strings("\n\nCool beans of the day: ", w1156) -> (w1154:string)
                    n414 = Build Array(w1154) -> (w1155:string[])
                  }
                }
                n415 = local read "Det.P input #"() -> (w1139:i32)
                n416 = for {
                  tunnel: w1147 -> [w1181] mode=indexing
                  tunnel: [w1182] -> w1131 mode=indexing
                  tunnel: w1146 -> [w1175]
                  tunnel: [w1174] -> w1145 mode=indexing
                  n417 = Index Array(array=w1175, index=w1181) -> (element=w1174:dbl)
                  n418 = Format Into String(format string="%.0f", w1181) -> (resulting string=w1178:string)  [unwired: 2 in, 1 out]
                  n419 = Format Into String(format string="%.2f", w1174) -> (resulting string=w1176:string)  [unwired: 2 in, 1 out]
                  n420 = Concatenate Strings("\nCh: " ("format string"), w1178, ", Temp: " ("format string"), w1176, "°C." ("format string")) -> (w1182:string)
                }
                n421 = Array Size(array=w1145) -> (size(s)=w1150:i32)
                n422 = Add Array Elements(numeric array=w1145) -> (sum=w1151:dbl)
                n423 = Index Array(array=w1138, index=w1139) -> (element=w1136:dbl)
                n424 = Divide(x=w1151, y=w1150) -> (x/y=w1148:dbl)
                n425 = Format Into String(format string="%.3f", w1136) -> (resulting string=w1134:string)  [unwired: 2 in, 1 out]
                n426 = Format Into String(format string="%.2f", w1148) -> (resulting string=w1128:string)  [unwired: 2 in, 1 out]
                n427 = Select(t="ACTIVE!!!!!", s=w1129, f="inactive.") -> (s? t:f=w1141:string)
                n428 = Concatenate Strings("Hello, XAMS teammembers.", "\n\nThe alarm is currently ", w1141, "\n\nThe latest detector pressure is: ", w1134, " bar." ("format string"), "\nTemperatures inside the detector are:", w1131, "\nThe average detector temperature is ", w1128, "°C." ("format string"), "\n\nThank you for doing your best today, once again!\nRegards, SC.", w1118) -> (w1123:string)
                "Status email preview" <- w1123
                n429 = call "custom_email_program.vi"("mail server"="smtp.nikhef.nl", "return address"="return address", "message"=w1123, "subject ([No Subject])"="XAMS daily status email.", "Email Adresses"="Email Addresses") -> ("error out"=w1115:errorcluster)  [unwired: 6 in]
                n430 = Unbundle By Name(w1115) -> ("code"=→"Email error":i32, "source"=→"source":string)
                n431 = Get Date/Time In Seconds() -> (seconds since 1Jan1904=w1125:timestamp)
                n432 = To Double Precision Float(number=w1125) -> (double precision float=w1124:dbl)
              }
            }
          }
        }
        n433 = Decrement(x="Cycles to execute") -> (x-1=w283:dbl)
        n434 = Decrement(x=w283) -> (x-1=w282:dbl)
        n435 = Greater?(x=w266, y=w282) -> ()  [unwired: 1 out]
        n436 = Decrement(x="Clear data every N cycles") -> (x-1=w263:dbl)
        n437 = Greater?(x=w266, y=w263) -> (0:w265:bool)
        n438 = And(x="Auto-clear data?", y=w265) -> (x .and. y?=w268:bool)
        n439 = Or(x=w268, y="Clear data") -> (x .or. y?=w270:bool)
        n440 = case shown="False" w270 {
          tunnel: w281 -> [w311 _]
          tunnel: [w311 dbl[][] []] -> w280
          tunnel: w279 -> [w310 _]
          tunnel: [w310 w317] -> w278
          tunnel: w277 -> [w309 _]
          tunnel: [w309 w317] -> w276
          tunnel: w275 -> [w308 _]
          tunnel: [w308 w315] -> w274
          tunnel: w273 -> [w307 _]
          tunnel: [w307 w313] -> w272
          tunnel: w266 -> [w306 _]
          tunnel: [w306 0] -> w267
          frame False {
          }
          frame True {
            w317 = 0.0
            n441 = Get Date/Time In Seconds() -> (seconds since 1Jan1904=w314:timestamp)
            n442 = To Double Precision Float(number=w314) -> (double precision float=w316:dbl)
            n443 = Build Array(w314) -> (w313:timestamp[])
            n444 = Build Array(w316, w316) -> (w315:dbl[])
          }
        }
        n445 = Or(x=FALSE, y="stop") -> (x .or. y?=w303:bool)
        "Auto-clear" <- "Auto-clear data?"
      }
    }
    frame True {
    }
  }
  n446 = flat-sequence {
    tunnel: w19 -> [w1226]
    tunnel: w15 -> [w1217]
    tunnel: w14 -> [w1214]
    tunnel: w13 -> [w1209]
    tunnel: w6 -> [w1198]
    tunnel: w1 -> [w1195]
    frame #0 {
      w1222 = u16 2 items=["1"=1, "2"=2] ("Heater Output (1:1)")
      w1223 = u16 0 items=["Off", "Low (On)", "Medium", "High"] ("Range (0:Off)")
      # "Important icons! Always press STOP button when done \ninstead of force closing, otherwise these don't get executed"
      # "Turn off heater, shutdown COM"
      # "Error Handling and Post-Processing (EHaPP)"
      n447 = Unbundle(w1226) -> ("VISA resource name out"=w1225:refnum<visa-resource-name>, "error out"=w1224:errorcluster)
      n448 = Unbundle(w1217) -> ("VISA resource name out"=w1216:refnum<visa-resource-name>, "error out"=w1215:errorcluster)
      n449 = Unbundle(w1214) -> ("VISA resource name out"=w1213:refnum<visa-resource-name>, "error out"=w1212:errorcluster)
      n450 = Unbundle(w1209) -> ("task out"=w1207:refnum<k21>, "error out"=w1205:errorcluster)
      n451 = Unbundle(w1198) -> ("task out"=w1202:refnum<k21>, "error out"=w1200:errorcluster)
      n452 = Unbundle(w1195) -> ("task out"=w1194:refnum<k21>, "error out"=w1193:errorcluster)
      n453 = call <vilib>:"DAQmx Stop Task.vi"("task/channels in"=w1207, "error in"=w1205) -> ("task out"=w1206:refnum<k21>, "error out"=w1204:errorcluster)  [unwired: 12 in]
      n454 = call <vilib>:"DAQmx Stop Task.vi"("task/channels in"=w1202, "error in"=w1200) -> ("task out"=w1201:refnum<k21>, "error out"=w1199:errorcluster)  [unwired: 12 in]
      n455 = call <vilib>:"DAQmx Stop Task.vi"("task/channels in"=w1194, "error in"=w1193) -> ("task out"=w1192:refnum<k21>, "error out"=w1196:errorcluster)  [unwired: 12 in]
      n456 = call <instrlib>:"Configure Output Range and Manual Value.vi"("VISA resource name"=w1225, "Heater Output (1:1)"=w1222, "Range (0:Off)"=w1223, "Manual Output (0.00 %)"=0.0, "error in (no error)"=w1224) -> ("VISA resource name out"=w1220:refnum<visa-resource-name>, "error out"=w1219:errorcluster)  [unwired: 9 in]
      n457 = call <instrlib>:"Close.vi"("error in (no error)"=w1215, "VISA resource name"=w1216) -> ("error out"=w1211:errorcluster)  [unwired: 9 in]
      n458 = call <instrlib>:"Close.vi"("error in (no error)"=w1212, "VISA resource name"=w1213) -> ("error out"=w1210:errorcluster)  [unwired: 9 in]
      n459 = call <instrlib>:"Close.vi"("error in (no error)"=w1219, "VISA resource name"=w1220) -> ("error out"=w1218:errorcluster)  [unwired: 9 in]
      n460 = call <vilib>:"DAQmx Clear Task.vi"("task in"=w1206, "error in"=w1204) -> ("error out"=w1208:errorcluster)  [unwired: 13 in]
      n461 = call <vilib>:"DAQmx Clear Task.vi"("task in"=w1201, "error in"=w1199) -> ("error out"=w1203:errorcluster)  [unwired: 13 in]
      n462 = call <vilib>:"DAQmx Clear Task.vi"("task in"=w1192, "error in"=w1196) -> ("error out"=w1197:errorcluster)  [unwired: 13 in]
      n463 = call <vilib>:"Simple Error Handler.vi"("error in (no error)"=w1218) -> ()  [unwired: 4 in, 5 out]
      n464 = call <vilib>:"Simple Error Handler.vi"("error in (no error)"=w1211) -> ()  [unwired: 4 in, 5 out]
      n465 = call <vilib>:"Simple Error Handler.vi"("error in (no error)"=w1210) -> ()  [unwired: 4 in, 5 out]
      n466 = call <vilib>:"Simple Error Handler.vi"("error in (no error)"=w1208) -> ()  [unwired: 4 in, 5 out]
      n467 = call <vilib>:"Simple Error Handler.vi"("error in (no error)"=w1203) -> ()  [unwired: 4 in, 5 out]
      n468 = call <vilib>:"Simple Error Handler.vi"("error in (no error)"=w1197) -> ()  [unwired: 4 in, 5 out]
    }
  }
  n469 = Array Size(array=w29) -> (size(s)=w32:i32)
  n470 = Decrement(x=w32) -> (x-1=w31:i32)
  n471 = Index Array(array=w29, index #1=w31, index #2=1 ("index")) -> (element #1=w30:timestamp, element #2=w11:timestamp)
  n472 = To Double Precision Float(number=w30) -> (double precision float=w28:dbl)
  n473 = To Double Precision Float(number=w11) -> (double precision float=w27:dbl)
  n474 = Subtract(x=w28, y=w27) -> ()  [unwired: 1 out]
  "Started up?" <- w23
